vi "ER2007 Test Panel.vi"() -> ()   [LabVIEW 2013]
uses:
  Controls/Global ER2007.vi
panel:
  in  "Defeated":bool
  in  "Sim":bool
  in  "Radio Cell Selects":T1(ring)
  out "Clock":string
  in  "Reset DAQ":bool
  out "VPA Err":bool
  out "Elap-T":string="Lapsed Hrs"
  out "Last-T":string="Time"
  out "ProdVol":string="Produced Vol (cc)"
  out "Dnstrm-P":string="Downstrm P (psi)"
  out "Delta-P":string="Delta-P (psi)"
  out "Pore-P":string="Pore P (psi)"
  out "Conf-P":string="Confining P (psi)"
  out "TB":string="T-B (°C)"
  out "TA":string="T-A (°C)"
  out "FF23":string="FF 2-3"
  out "ER23":string="E-R 2-3 (Ohm-m)"
  out "ER14":string="E-R 1-4 (Ohm-m)"
  out "ER13":string="E-R 1-3 (Ohm-m)"
  out "ER12":string="E-R 1-2 (Ohm-m)"
  out "SampID":string="Sample ID"
  out "Cell #":string="Cell #"
  out "Status":string="Status"
  out "Other PC Busy":bool
  out "GCD Reset":bool
  out "Delta P (psi)":dbl[](array[numeric]) format="%.2f"
  out "Pc-d(psig)":dbl[](array[numeric])
  in  "TakePt":bool
  out "System Error":bool
  out "Refresh":bool
  out "SetupCell":i32
  out "GCDCell":i32
  out "SelCell":i32
  out "C5-Status":bool caption="VPA"
  out "C4-Status":bool caption="Manual"
  out "C3-Status":bool caption="VPA"
  out "C2-Status":bool caption="Manual"
  out "C1-Status":bool caption="Manual"
  in  "GCD Progress Titles":string="Initialize  Main Eng  Determ-R  Final Vals Close HP Close NAII"
  out "GCD Prog":bool[](array[boolean])
  out "Selected Data Cell":i32
  out "Cell Data Idx":i32
  out "Cur Time":dbl
  out "Schd Times":dbl[](array[numeric])
  out "GCD Err":bool
  out "GCD Busy":bool
  out "A/D Err":bool
  out "DAQ Run":bool
  in  "Radio Cell Selects":T2(radio)
  in  "Utilities":bool
  out "F 2-3":dbl[](array[numeric])=[6.3872, 0.0, 5.0918, 5.4196, 0.0, 5.8365, 5.8365, 0.0] format="%.2f"
  out "Cell":string[](array[string])=["Cell 1", "Cell 2", "Cell 3", "Cell 4", "Cell 5", "Cell 6B", "6B", "6C"]
  out "Copyrightl":string="Program ER2005, Version 1.00, DCI Inc, Copyright 2005, All Rights Reserved"
  out "Disp Pv (ml)":dbl[](array[numeric])=[12.345, 0.0, 2.509, 2.736, 0.0, 1.983, 508.0, 0.0] format="%.2f"
  in  "CurVals":bool
  in  "History":bool
  in  "Setup":bool
  in  "Stop":bool
  out "Lapsed Hrs":dbl[](array[numeric])=[789.0, 0.0, 107.6, 105.8, 0.0, 51.2, 51.2, 0.0] format="%.1f"
  out "Time":timestamp[](array[timestamp])=[timestamp(3199615260.25 s since 1904-01-01), timestamp(3199586400.25 s since 1904-01-01), timestamp(3199635000.25 s since 1904-01-01), timestamp(3199623780.25 s since 1904-01-01), timestamp(3199586400.25 s since 1904-01-01), timestamp(3199669020.25 s since 1904-01-01), timestamp(3199669020.25 s since 1904-01-01), timestamp(3199586400.25 s since 1904-01-01)] format="%<%H:%M>T"
  out "Pc (psig)":dbl[](array[numeric])=[7492.0, 0.0, 3520.0, 3488.0, 0.0, 508.0, 508.0, 0.0]
  out "NOP (psig)":dbl[](array[numeric])=[10058.0, 0.0, 5018.0, 4993.0, 0.0, 904.0, 904.0, 0.0]
  out "T-B (°C)":dbl[](array[numeric])=[149.0, 23.0, 153.0, 149.0, 23.0, 150.0, 150.0, 22.0] format="%.1f"
  out "T-A (°C)":dbl[](array[numeric])=[152.0, 22.0, 150.0, 147.0, 23.0, 151.0, 151.0, 22.0] format="%.1f"
  out "ER 2-3":dbl[](array[numeric])=[6.3872, 0.0, 5.0918, 5.4196, 0.0, 5.8365, 5.8365, 0.0] format="%.3f"
  out "ER 1-4":dbl[](array[numeric])=[6.1683, 0.0, 5.0447, 5.2485, 0.0, 5.6703, 5.6703, 0.0] format="%.3f"
  out "ER 1-3":dbl[](array[numeric])=[6.0887, 0.0, 4.9169, 5.2753, 0.0, 5.5338, 5.5338, 0.0] format="%.3f"
  out "ER 1-2":dbl[](array[numeric])=[6.7304, 0.0, 5.356, 5.9831, 0.0, 6.0646, 6.0646, 0.0] format="%.3f"
  out "Sample ID":string[](array[string])=["Sample #1", "", "Sample #3", "Sample #4", "", "Sample #6", "Sample #6", "  "]
  out "Status":bool[](array[boolean])=[FALSE, FALSE, FALSE, FALSE, FALSE, FALSE, TRUE, FALSE]
  # "Test Data"
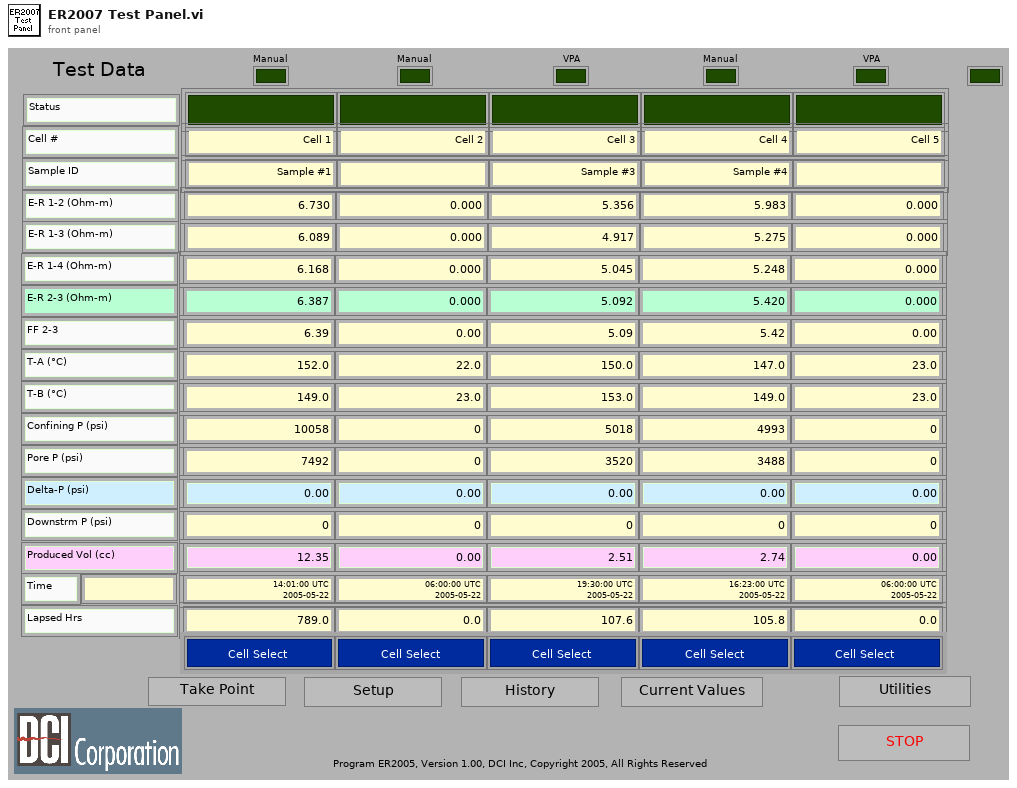
[diagram p1: front panel]
types:
  T1 = enum32{"No Selection", "CS 1", "CS 2", "CS 3", "CS 4", "CS 5", "CS 6"}
  T2 = enum32{"No Selection", "CS 1", "CS 2", "CS 3", "CS 4", "CS 5"}
  T3 = cluster{"PageTitle":string, "NumLines":i32, "ChlNum":string[], "ChlDesc":string[], "ChlUnits":string[], "ChlZero":sgl[], "ChlFactor":sgl[], "ChlConfig":u16[]}[]
  T4 = enum16{"Cell 1", "Cell 2", "Cell 3", "Cell 4", "Cell 5", "Cell 6A", "Cell 6B", "Cell 6C"}[]
  T5 = cluster{"CurCell":i32, "Cell Data":cluster{"Cell ID":i32, "Cell Status":enum16{"Inactive", "Setup", "Active", "Done"}, "Project":string, "Sample #":string, "Rock Type":string, "Fluid Pair":string, "Rw":dbl, "Rw Temp":dbl, "Length":dbl, "Diameter":dbl, "Porosity":dbl, "Permeability":dbl, "4P":bool, "ElectSpace":dbl, "Frequency":dbl, "Amplitude":dbl, "DAQ Period":u32, "DAQ Units":u16, "Start Time":dbl, "Next Time":dbl, "Datafile":path, "Last Pore Vol":dbl, "Last Pore Xdcr":enum16{"<none>", "Lo Range", "Hi Range"}, "Last Resistor":enum16{"<none>", "Resistor 1", "Resistor 2", "Resistor 3", "Resistor 4", "Resistor 5", "Resistor 6"}, "CurData":dbl[][], "Comment":string}[]}
  T6 = cluster{"Cell ID":i32, "Cell Status":enum16{"Inactive", "Setup", "Active", "Done"}, "Project":string, "Sample #":string, "Rock Type":string, "Fluid Pair":string, "Rw":dbl, "Rw Temp":dbl, "Length":dbl, "Diameter":dbl, "Porosity":dbl, "Permeability":dbl, "4P":bool, "ElectSpace":dbl, "Frequency":dbl, "Amplitude":dbl, "DAQ Period":u32, "DAQ Units":u16, "Start Time":dbl, "Next Time":dbl, "Datafile":path, "Last Pore Vol":dbl, "Last Pore Xdcr":enum16{"<none>", "Lo Range", "Hi Range"}, "Last Resistor":enum16{"<none>", "Resistor 1", "Resistor 2", "Resistor 3", "Resistor 4", "Resistor 5", "Resistor 6"}, "CurData":dbl[][], "Comment":string}[]
  T7 = cluster{"Cell ID":i32, "Cell Status":enum16{"Inactive", "Setup", "Active", "Done"}, "Project":string, "Sample #":string, "Rock Type":string, "Fluid Pair":string, "Rw":dbl, "Rw Temp":dbl, "Length":dbl, "Diameter":dbl, "Porosity":dbl, "Permeability":dbl, "4P":bool, "ElectSpace":dbl, "Frequency":dbl, "Amplitude":dbl, "DAQ Period":u32, "DAQ Units":u16, "Start Time":dbl, "Next Time":dbl, "Datafile":path, "Last Pore Vol":dbl, "Last Pore Xdcr":enum16{"<none>", "Lo Range", "Hi Range"}, "Last Resistor":enum16{"<none>", "Resistor 1", "Resistor 2", "Resistor 3", "Resistor 4", "Resistor 5", "Resistor 6"}, "CurData":dbl[][], "Comment":string}
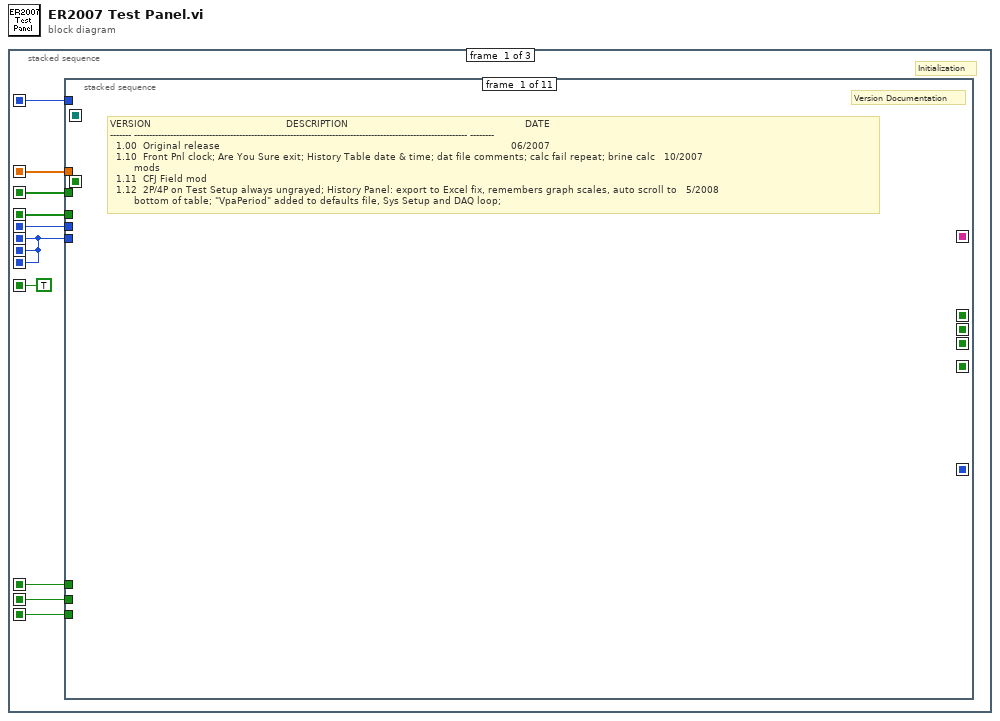
[diagram p0: block diagram]
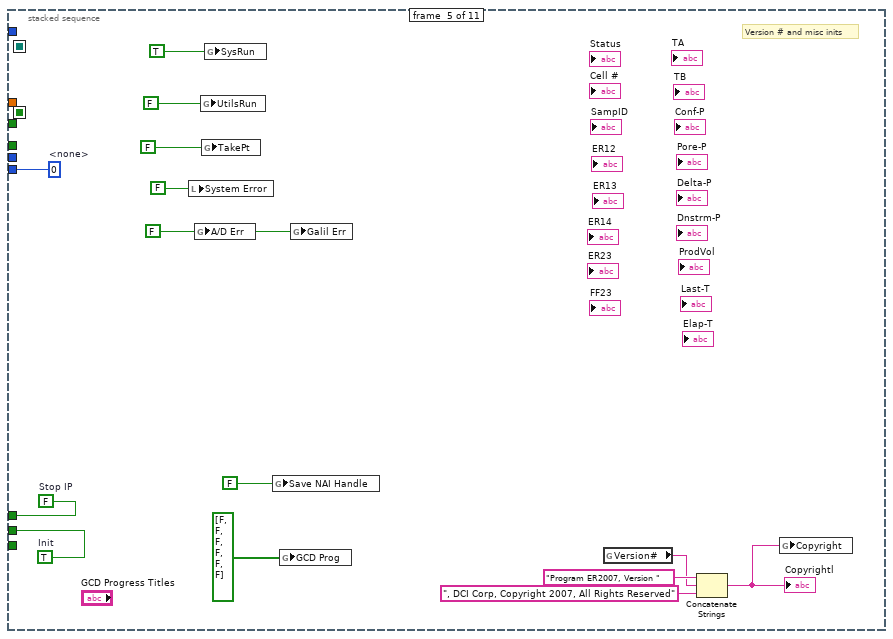
[diagram p5: hidden frame]
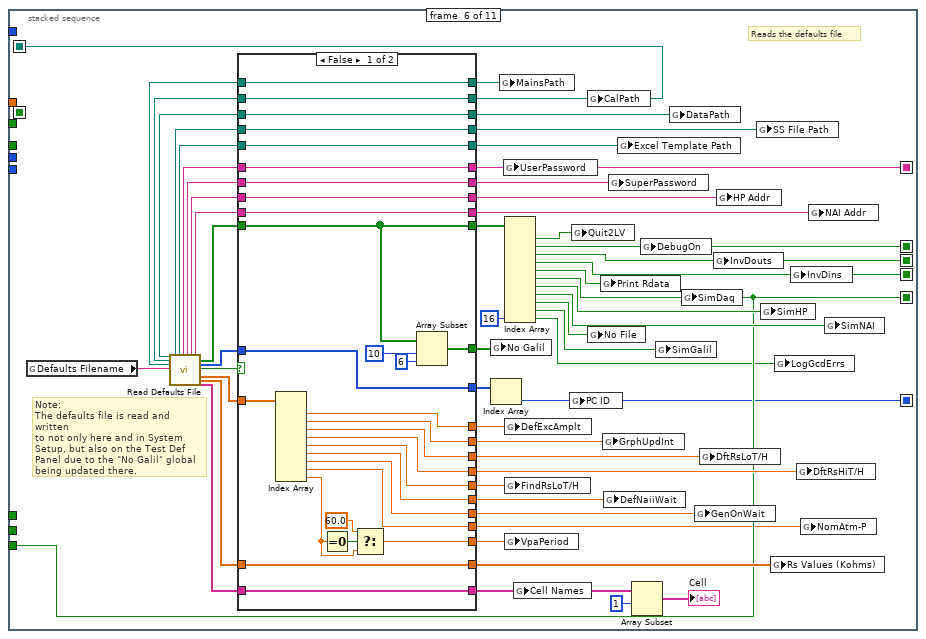
[diagram p6: hidden frame]
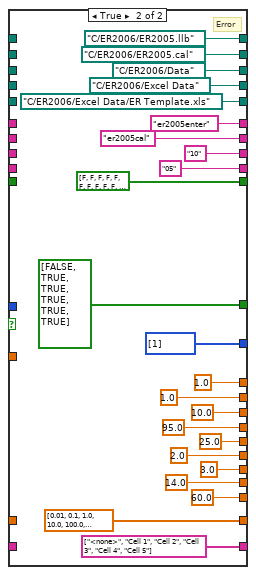
[diagram p7: hidden frame]
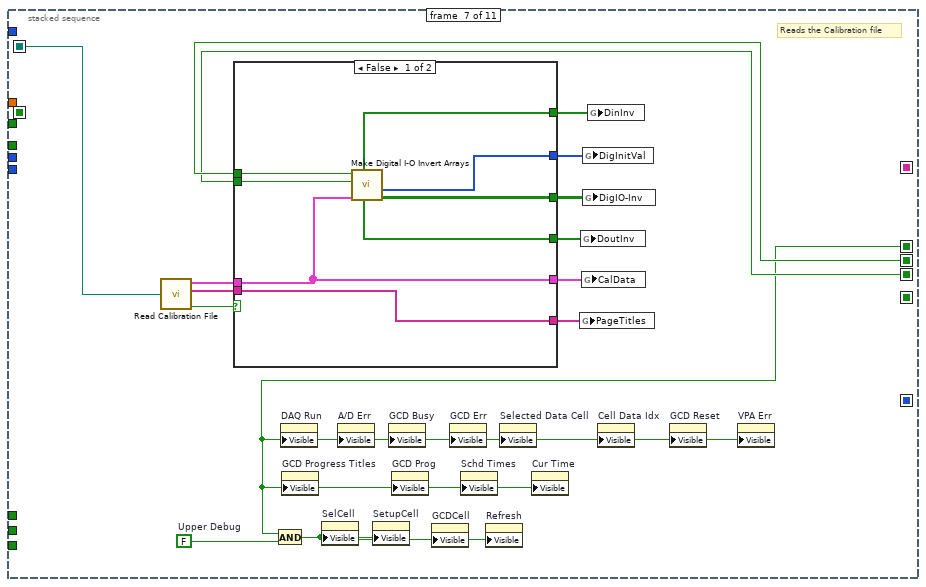
[diagram p8: hidden frame]
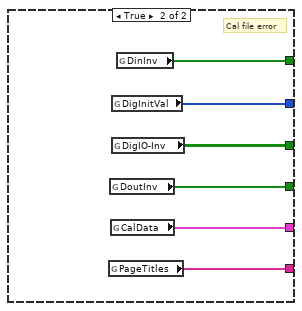
[diagram p9: hidden frame]
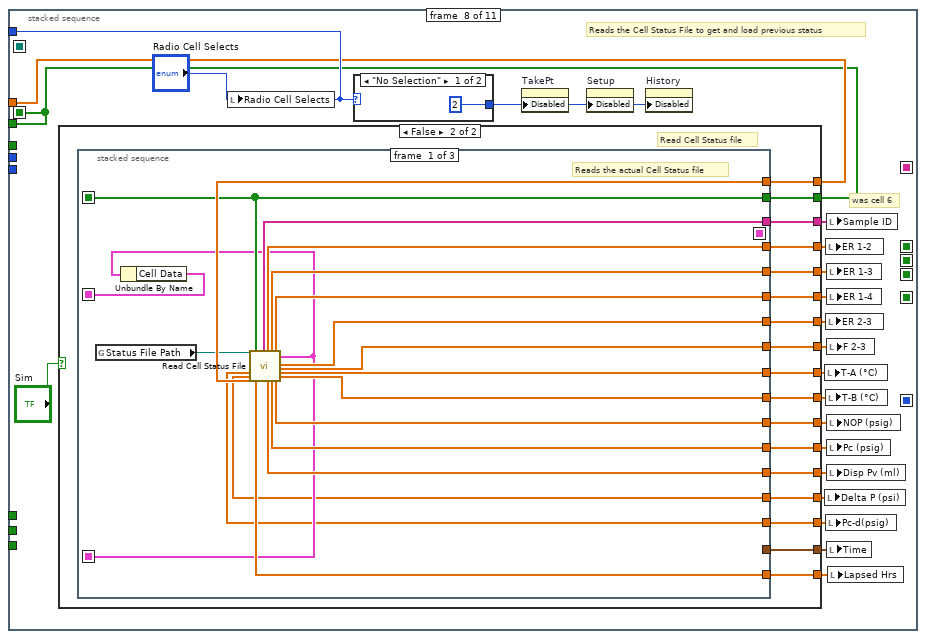
[diagram p10: hidden frame]
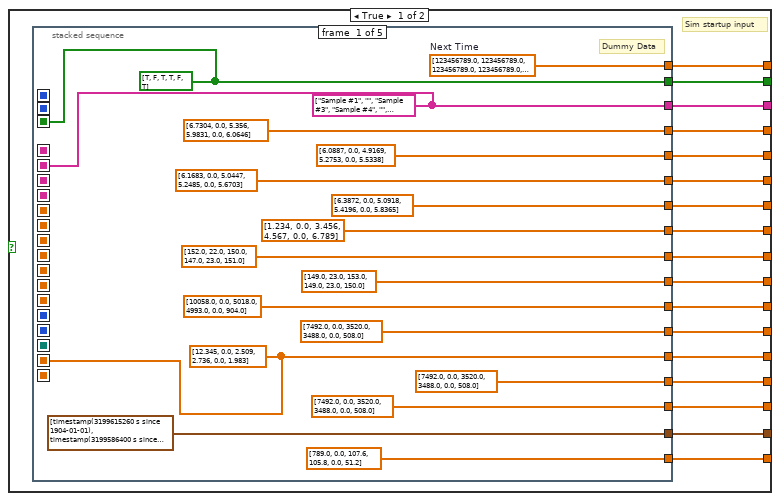
[diagram p11: hidden frame]
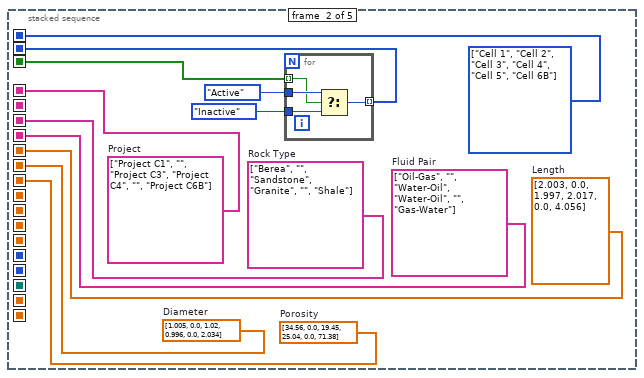
[diagram p12: hidden frame]
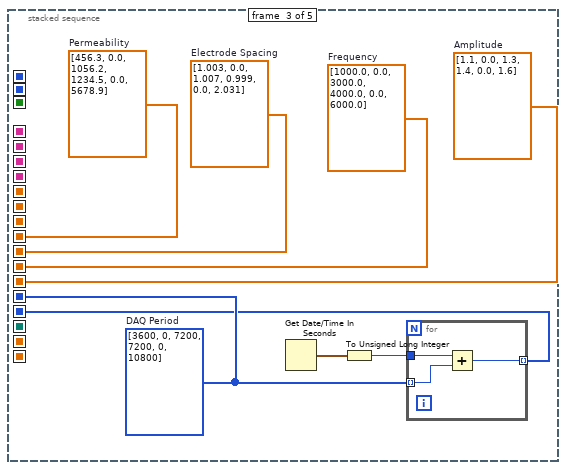
[diagram p13: hidden frame]
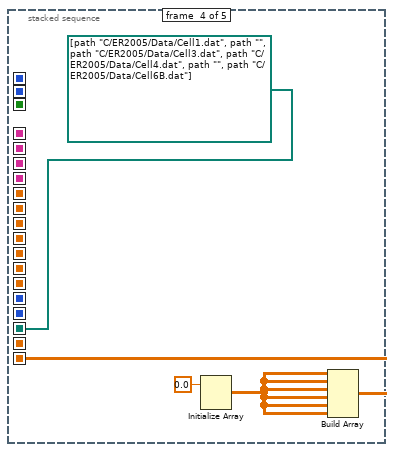
[diagram p14: hidden frame]
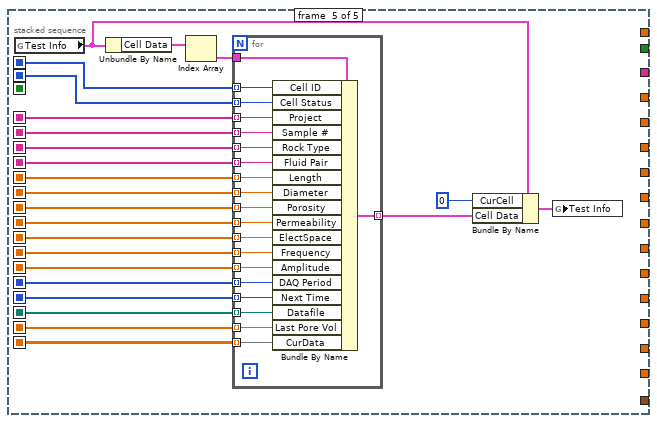
[diagram p15: hidden frame]
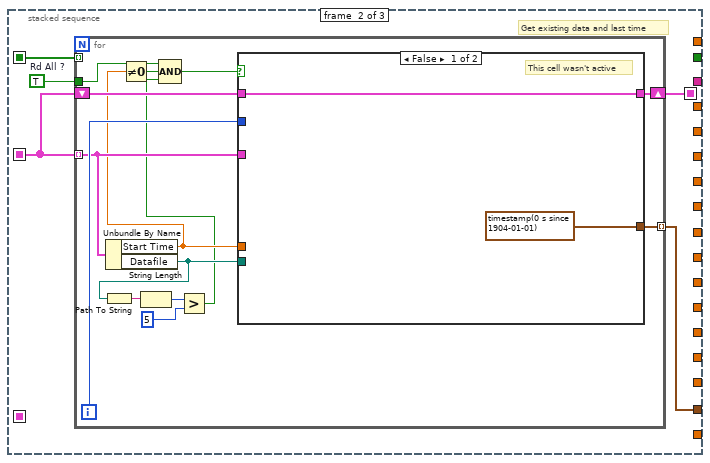
[diagram p16: hidden frame]
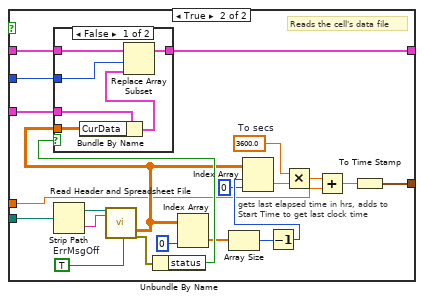
[diagram p17: hidden frame]
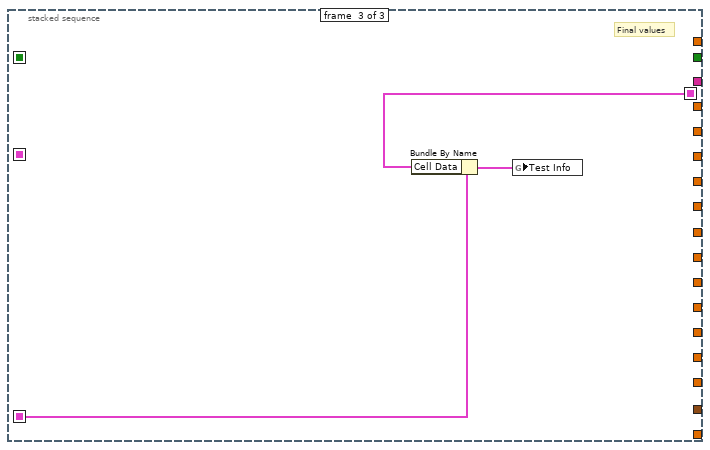
[diagram p19: hidden frame]
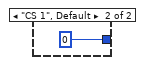
[diagram p20: hidden frame]
diagram:
  n1 = stacked-sequence {
    seq-local: [w10 _ _] -> [_ w451 _]
    seq-local: [w9 _ _] -> [_ w450 _]
    seq-local: [w8 _ _] -> [_ w449 _]
    seq-local: [w7 _ _] -> [_ w448 _]
    seq-local: [w6 _ _] -> [_ w447 _]
    seq-local: [w5 _ _] -> [_ w445 _]
    seq-local: [w5 _ _] -> [_ w446 _]
    seq-local: [w5 _ _] -> [_ w444 _]
    seq-local: [TRUE _ _] -> [_ w443 _]
    seq-local: [w3 _ _] -> [_ w442 w1331]
    seq-local: [w2 _ _] -> [_ w441 _]
    seq-local: [w1 _ _] -> [_ w440 _]
    frame #0 {
      # "Initialization"
      n2 = stacked-sequence {
        seq-local: [_ _ _ _ _ w58 _ _ _ _ _] -> [_ _ _ _ _ _ w140 _ _ _ _]
        seq-local: [_ _ _ _ _ w57 _ _ _ _ _] -> [_ _ _ _ _ _ _ _ _ _ _]
        seq-local: [_ _ _ _ _ w52 _ _ _ _ _] -> [_ _ _ _ _ _ w142 _ _ _ _]
        seq-local: [_ _ _ _ _ w53 _ _ _ _ _] -> [_ _ _ _ _ _ w141 _ _ _ _]
        seq-local: [_ _ _ _ _ _ _ w162 _ _ _] -> [_ _ _ _ _ _ _ _ _ w391 _]
        seq-local: [_ _ _ _ _ w50 _ _ _ _ _] -> [_ _ _ _ _ _ w131 _ _ _ _]
        seq-local: [_ _ _ _ _ w35 _ _ _ _ _] -> [_ _ _ _ _ _ _ _ w383 _ _]
        seq-local: [_ _ _ _ _ w34 _ _ _ _ _] -> [_ _ _ _ _ _ _ _ w380 _ _]
        tunnel: [_ _ _ _ _ _ _ w164 _ _ _] -> w10
        tunnel: [_ _ _ _ _ _ _ "Radio Cell Selects" _ _ _] -> w9
        tunnel: [_ _ _ _ w22 _ _ _ _ _ _] -> w8
        tunnel: [_ _ _ _ _ _ _ w162 _ _ _] -> w7
        tunnel: [_ _ _ _ _ _ _ _ _ w388 _] -> w6
        tunnel: [_ _ _ _ w13 _ _ _ _ _ _] -> w5
        tunnel: [_ _ _ _ _ w35 _ _ _ _ _] -> w3
        tunnel: [_ _ _ _ _ _ _ _ w379 _ _] -> w2
        tunnel: [_ _ _ _ w11 _ _ _ _ _ _] -> w1
        frame #0 {
          # "VERSION                                             DESCRIPTION                                                           DATE \n------- --------------------------------------------------------------------------------------------------------------- --------\n  1.00  Original release                                                                                                 06/2007\n  1.10  Front Pnl clock; Are You Sure exit; History Table date & time; dat file comments; calc fail repeat; brine calc   10/2007\n        mods\n  1.11  CFJ Field mod\n  1.12  2P/4P on Test Setup always ungrayed; History Panel: export to Excel fix, remembers graph scales, auto scroll to   5/2008\n        bottom of table; \"VpaPeriod\" added to defaults file, Sys Setup and DAQ loop;"
          # "Version Documentation"
        }
        frame #1 {
          # "New Cell Status Format\n\n[GenInfo]\nTitle=\"Cell Status Data File\"\nVersion=1.00\nLast Write=8/7/2005\nCurCell=\"2\"\n*NumCells=\"5\"\n[Cell 1 Status]\nCell ID=\"Cell 1\"\nStatus=Inactive\nProject=\"Project Cell 1\"\nSample ID=\"Sample #1\"\nRock Type=Granite\nFluid Pair=\"Brine & Air\"\nRw=11.000000\nRw Temp=22.000000\nLength=5.080000\nDiameter=2.540000\nPorosity=33.000000\nPermeability=8.000000\n2P/4P=4P\nElect Spacing=2.540000\nFrequency=1000.000000\nAmplitude=1.000000\nDAQ Period=1\nDAQ Units=Hrs\nStart Time=3205931570.670000\nNext Time=3205935200.670000\nFilename=\"C:\\\\ER2005\\\\Data\\\\Cell 1 Data.dat\"\nPore Volume=1.000000\n*Pore Transducer=\"Lo Range\"\nLast Resistor=\"Resistor 5\"\nER 1-2=4023.631104\nER 1-3=2923.760010\nER 1-4=3594.040039\nER 2-3=2434.518066\nFF 2-3=235.399994\nTemp A=24.799999\nTemp B=24.799999\nConf Press=5.000000\nPore Press=2.330000\nDelta-Press=\nPore-Down=\n[Cell 2 Status]"
          # "New Data File Format-Data Line\n\n                        Reals\nCol #  Process Variable Col #\n----- ----------------- -----\n  1   Point Flag\n  2   Point Date\n  3   Point Time\n  4   Elapsed Time (hrs)   1\n  5   ER 1-2               2\n  6   ER 1-3               3\n  7   ER 1-4               4\n  8   ER 2-3               5\n  9   F 2-3                6\n 10   T-A                  7\n 11   T-B                  8\n 12   Conf P (ER2005 NOP)  9\n 13   Pore P (ER2005 Pc)  10\n 14   Delta-P             11\n 15   Downstrm P (Pc-d)   12\n 16   Produced Vol        13\n 17   C14                 14\n 18   C23                 15\n 19   Comment"
          # "Dynamically Launched vi's:                     Other Required Files: simply copy them to System32\n-----------------------------------------      --------------------------------------------------------\nER2007 Are You Sure Popup Panel.vi             C:\\Windows\\System32\\instrsup.dll - used by NAII vi's\nER2007 Background DAQ Loop.vi                  C:\\Windows\\System32\\NAI2250.dll - used by NAII vi's\nER2007 Calibration Panel.vi                    C:\\Windows\\System32\\DMC32.dll - used by Galil vi's\nER2007 Current Values Panel.vi                 \nER2007 Data History Panel.vi\nER2007 Get Cell Data.vi\nER2007 Maintenance Panel.vi\nER2007 Password Popup Panel.vi\nER2007 System Setup Panel.vi\nER2007 Take Data Popup Panel.vi\nER2007 Test Definition Panel.vi\nER2007 Utilities Menu Panel.vi\nC:\\Program Files\\National Instruments\\LabVIEW 7.1\\vi.lib\\\n (cont)  addons\\_office\\_exclsub.llb\\_Excel Dynamic VIs.vi"
          # "Data File Format-Header\n\nStart Date\nStart Time\nFilename\nProject\nSample ID\nRock Type\nFluid Pair\nRw\nRt\nFrequency\nAmplitude\nDAQ Period (mins)\nLength\nDiameter\nPorosity\nPermeability\nElectrode Spacing"
          # "The arrays and controls on the front panel are a Arial Bold at 20 pt (18 pt plus two cntrl+)\nThe front panel color (matches Logo): Hue-135; Sat-43; Lum-109; Red-95; Grn-121; Blue-137"
          # "Notes and misc initilization"
        }
        frame #2 {
          # "More notes: Device 1 hardware assignments"
          # "PCI-6220 PV Assignments\n\n                      Connector 0\n        DIGITAL OUTS                ANALOG INS\n----------------------------  ------------------------\nP0.0    Shunt NOP1/Pc1A       AI 0    NOP1\nP0.1    SCL1                  AI 1    TC1A\nP0.2    SCL2                  AI 2    TC1B\nP0.3    Shunt Pc1B            AI 3    Pc1B\nP0.4    Auto Enable           AI 4    <spare>\nP0.5    RSCL1                 AI 5    <spare>\nP0.6    <spare>               AI 6    <spare>\nP0.7    RSCL2                 AI 7    <spare>\n\nP1.0    RSCL3                 AI 8    Pc1A\nP1.1    YCL1                  AI 9    CJ1A\nP1.2    YCL2                  AI 10   CJ1B\nP1.3    YCL3                  AI 11   <spare>\nP1.4    YCL4                  AI 12   <spare>\nP1.5    <spare>               AI 13   <spare>\nP1.6    Lockout               AI 14   <spare>\nP1.7    <spare>               AI 15   <spare>\n\n        DIGITAL INS\n----------------------------\nP2.0    <spare>\nP2.1    <spare>\nP2.2    <spare>\nP2.3    <spare>\nP2.4    <spare>\nP2.5    <spare>\nP2.6    <spare>\nP2.7    <spare>"
        }
        frame #3 {
          # "GPIB Setup and Operational Notes\n\n1) Using MAX, setup the PC #1 GPIB board as System\n   Controller with a primary address of 1.  Setup the\n   PC #2 GBIP board as a Non-System Controller with a\n   primary address of 2.\n2) Initialization is still a problem\n3) When PC #1 is active (taking a point), it asserts\n   Send IFC to clear the bus and take charge.  After\n   it has completed, it returns CIC control to PC #2\n   using PassControl."
          # "PCI-6224 PV Assignments By Connector Number\n\n                      Connector 1\n        DIGITAL OUTS                ANALOG INS\n----------------------------  ------------------------\nP0.8    Shunt NOP4/Pc4A       AI 16   NOP4\nP0.9    <spare>               AI 17   TC4A\nP0.10   <spare>               AI 18   TC4B\nP0.11   Shunt NOP5/Pc4B       AI 19   Pc4B\nP0.12   <spare>               AI 20   <spare>\nP0.13   Shunt Pc5A/Pc5B       AI 21   Pc5A\nP0.14   <spare>               AI 22   TC5A\nP0.15   <spare>               AI 23   TC5B\n\n                              AI 24   Pc4A\n                              AI 25   CJ4A\n                              AI 26   CJ4B\n                              AI 27   NOP5\n                              AI 28   <spare>\n                              AI 29   Pc5B\n                              AI 30   CJ5A\n                              AI 31   CJ5B"
          # "PCI-6224 PV Assignments By Connector Number\n\n                      Connector 0\n        DIGITAL OUTS                ANALOG INS\n----------------------------  ------------------------\nP0.0    Shunt NOP2/Pc2A       AI 0    NOP2\nP0.1    <spare>               AI 1    TC2A\nP0.2    <spare>               AI 2    TC2B\nP0.3    Shunt NOP3/Pc2B       AI 3    Pc2B\nP0.4    <spare>               AI 4    <spare>\nP0.5    Shunt Pc3A/Pc3B       AI 5    Pc3A\nP0.6    <spare>               AI 6    TC3A\nP0.7    <spare>               AI 7    TC3B\n\nP1.0    <spare>               AI 8    Pc2A\nP1.1    <spare>               AI 9    CJ2A\nP1.2    <spare>               AI 10   CJ2B\nP1.3    <spare>               AI 11   NOP3\nP1.4    <spare>               AI 12   <spare>\nP1.5    <spare>               AI 13   Pc3A\nP1.6    <spare>               AI 14   CJ3A\nP1.7    <spare>               AI 15   CJ3B\n\n        DIGITAL INS\n----------------------------\nP2.0    Busy 1\nP2.1    Busy 2\nP2.2    <spare>\nP2.3    <spare>\nP2.4    <spare>\nP2.5    <spare>\nP2.6    <spare>\nP2.7    <spare>"
          # "More notes: Device 2 hardware assignments"
        }
        frame #4 {
          w11 = FALSE  # Stop IP
          w12 = FALSE ("A/D Err")
          w13 = 0  # <none>
          w22 = TRUE  # Init
          # "Version # and misc inits"
          n3 = local write "System Error"(FALSE ("System Error")) -> ()
          n4 = global write "Global ER2007.vi" "A/D Err"(w12) -> ()
          n5 = global write "Global ER2007.vi" "UtilsRun"(FALSE ("UtilsRun")) -> ()
          n6 = global write "Global ER2007.vi" "TakePt"(FALSE ("New Setup")) -> ()
          n7 = global write "Global ER2007.vi" "SysRun"(TRUE ("SysRun")) -> ()
          n8 = global write "Global ER2007.vi" "Save NAI Handle"(FALSE ("Save NAI Handle")) -> ()
          n9 = global write "Global ER2007.vi" "GCD Prog"(bool[] [FALSE, FALSE, FALSE, FALSE, FALSE, FALSE] ("GCD Prog")) -> ()
          n10 = global write "Global ER2007.vi" "Galil Err"(w12) -> ()
          n11 = global read "Global ER2007.vi" "Version#"() -> (w20:string)
          n12 = Concatenate Strings("Program ER2007, Version " ("Substring"), w20, ", DCI Corp, Copyright 2007, All Rights Reserved" ("Substring")) -> (w19:string)
          "Copyrightl" <- w19
          n13 = global write "Global ER2007.vi" "Copyright"(w19) -> ()
        }
        frame #5 {
          # "Note:\nThe defaults file is read and written\nto not only here and in System\nSetup, but also on the Test Def\nPanel due to the \"No Galil\" global\nbeing updated there."
          # "Reads the defaults file"
          n14 = global read "Global ER2007.vi" "Defaults Filename"() -> (w37:string)
          n15 = call "Read Defaults File.vi"("Filename"=w37) -> ("DirPath3"=w73:path, "DirPath2"=w74:path, "DirPath1"=w75:path, "DirPath4"=w66:path, "DirPath5"=w65:path, "String1"=w72:string, "String2"=w71:string, "String3"=w69:string, "String4"=w68:string, "BooleanArray"=w77:bool[], "IntegerArray1"=w64:i32[], "ErrOut"=w78:bool, "RealArray1"=w70:dbl[], "RealArray2"=w67:dbl[], "StringArray"=w36:string[])  [unwired: 12 out]
          n16 = case shown="False" w78 {
            tunnel: w77 -> [w86 _]
            tunnel: [w86 bool[] [FALSE, FALSE, FALSE, FALSE, FALSE, FALSE, FALSE, FALSE, FALSE, FALSE, FALSE, FALSE] ("BooleanArray")] -> w76
            tunnel: [w107 path "C:/ER2006/ER2005.llb" ("DirPath1")] -> w59
            tunnel: w75 -> [w107 _]
            tunnel: [w106 path "C:/ER2006/ER2005.cal" ("DirPath2")] -> w58
            tunnel: w74 -> [w106 _]
            tunnel: [w105 path "C:/ER2006/Data" ("DirPath3")] -> w62
            tunnel: w73 -> [w105 _]
            tunnel: [w104 "er2005enter" ("String1")] -> w57
            tunnel: w72 -> [w104 _]
            tunnel: [w103 "er2005cal" ("String2")] -> w56
            tunnel: w71 -> [w103 _]
            tunnel: w70 -> [w100 _]
            tunnel: [w102 "10" ("String3")] -> w55
            tunnel: w69 -> [w102 _]
            tunnel: [w101 "05" ("String4")] -> w54
            tunnel: w68 -> [w101 _]
            tunnel: [w99 1.0] -> w45
            tunnel: [w98 1.0] -> w44
            tunnel: [w97 10.0] -> w43
            tunnel: [w96 95.0] -> w42
            tunnel: w67 -> [w95 _]
            tunnel: [w95 dbl[] [0.01, 0.1, 1.0, 10.0, 100.0, 1000.0] ("RealArray2")] -> w38
            tunnel: [w94 25.0] -> w41
            tunnel: [w93 path "C:/ER2006/Excel Data" ("SS File Path")] -> w61
            tunnel: w66 -> [w93 _]
            tunnel: [w92 2.0] -> w40
            tunnel: [w91 3.0] -> w39
            tunnel: [w90 path "C:/ER2006/Excel Data/ER Template.xls" ("Excel Template Path")] -> w60
            tunnel: w65 -> [w90 _]
            tunnel: w64 -> [w89 _]
            tunnel: [w89 i32[] [1] ("IntegerArray1")] -> w63
            tunnel: w36 -> [w88 _]
            tunnel: [w88 string[] ["<none>", "Cell 1", "Cell 2", "Cell 3", "Cell 4", "Cell 5"] ("StringArray")] -> w31
            tunnel: [w87 14.0 ("NomAtm-P")] -> w32
            tunnel: [w83 bool[] [FALSE, TRUE, TRUE, TRUE, TRUE, TRUE]] -> w28
            tunnel: [w79 60.0 ("VpaPeriod")] -> w25
            frame False {
              n17 = Index Array(array=w100) -> (element #1=w99:dbl, element #2=w98:dbl, element #3=w97:dbl, element #4=w96:dbl, element #5=w94:dbl, element #6=w92:dbl, element #7=w91:dbl, element #8=w87:dbl, element #9=w80:dbl)  [unwired: 9 in]
              n18 = Equal To 0?(x=w80) -> (x = 0?=w82:bool)
              n19 = Select(t=60.0, s=w82, f=w80) -> (s? t:f=w79:dbl)
              n20 = Array Subset(array=w86, index=10, length=6) -> (w83:bool[])
            }
            frame True {
              # "Error"
            }
          }
          n21 = global write "Global ER2007.vi" "No Galil"(w28) -> ()
          n22 = Index Array(array=w63) -> (element=w34:i32)  [unwired: 1 in]
          n23 = global write "Global ER2007.vi" "MainsPath"(w59) -> ()
          n24 = global write "Global ER2007.vi" "UserPassword"(w57) -> ()
          n25 = Index Array(array=w76, index #11=16 ("index")) -> (element #1=w51:bool, element #2=w50:bool, element #3=w52:bool, element #4=w53:bool, element #5=w49:bool, element #6=w35:bool, element #7=w48:bool, element #8=w47:bool, element #9=w46:bool, element #10=w33:bool, element #11=w26:bool)  [unwired: 10 in]
          n26 = global write "Global ER2007.vi" "DefExcAmplt"(w45) -> ()
          n27 = global write "Global ER2007.vi" "FindRsLoT/H"(w41) -> ()
          n28 = global write "Global ER2007.vi" "VpaPeriod"(w25) -> ()
          n29 = global write "Global ER2007.vi" "Cell Names"(w31) -> ()
          n30 = global write "Global ER2007.vi" "PC ID"(w34) -> ()
          n31 = global write "Global ER2007.vi" "Quit2LV"(w51) -> ()
          n32 = global write "Global ER2007.vi" "CalPath"(w58) -> ()
          n33 = global write "Global ER2007.vi" "No File"(w46) -> ()
          n34 = global write "Global ER2007.vi" "Print Rdata"(w49) -> ()
          n35 = global write "Global ER2007.vi" "GrphUpdInt"(w44) -> ()
          n36 = global write "Global ER2007.vi" "DefNaiiWait"(w40) -> ()
          n37 = global write "Global ER2007.vi" "SuperPassword"(w56) -> ()
          n38 = global write "Global ER2007.vi" "Excel Template Path"(w60) -> ()
          n39 = Array Subset(array=w31, index=1) -> (→"Cell":string[])  [unwired: 1 in]
          n40 = global write "Global ER2007.vi" "DebugOn"(w50) -> ()
          n41 = global write "Global ER2007.vi" "SimGalil"(w33) -> ()
          n42 = global write "Global ER2007.vi" "DataPath"(w62) -> ()
          n43 = global write "Global ER2007.vi" "SimDaq"(w35) -> ()
          n44 = global write "Global ER2007.vi" "GenOnWait"(w39) -> ()
          n45 = global write "Global ER2007.vi" "DftRsLoT/H"(w43) -> ()
          n46 = global write "Global ER2007.vi" "InvDouts"(w52) -> ()
          n47 = global write "Global ER2007.vi" "HP Addr"(w55) -> ()
          n48 = global write "Global ER2007.vi" "SS File Path"(w61) -> ()
          n49 = global write "Global ER2007.vi" "SimHP"(w48) -> ()
          n50 = global write "Global ER2007.vi" "Rs Values (Kohms)"(w38) -> ()
          n51 = global write "Global ER2007.vi" "LogGcdErrs"(w26) -> ()
          n52 = global write "Global ER2007.vi" "InvDins"(w53) -> ()
          n53 = global write "Global ER2007.vi" "DftRsHiT/H"(w42) -> ()
          n54 = global write "Global ER2007.vi" "NomAtm-P"(w32) -> ()
          n55 = global write "Global ER2007.vi" "NAI Addr"(w54) -> ()
          n56 = global write "Global ER2007.vi" "SimNAI"(w47) -> ()
        }
        frame #6 {
          w138 = FALSE  # Upper Debug
          # "Reads the Calibration file"
          n57 = call "Read Calibration File.vi"("Filepath"=w140) -> ("CalData"=w144:T3, "PageTitles"=w143:string[], "ErrOut"=w145:bool)  [unwired: 1 in, 2 out]
          n58 = case shown="False" w145 {
            tunnel: w144 -> [w152 _]
            tunnel: w143 -> [w153 _]
            tunnel: [w152 w154] -> w133
            tunnel: [w153 w155] -> w132
            tunnel: w142 -> [w151 _]
            tunnel: w141 -> [w150 _]
            tunnel: [w149 w156] -> w134
            tunnel: [w148 w157] -> w135
            tunnel: [w147 w158] -> w136
            tunnel: [w146 w159] -> w137
            frame False {
              n59 = call "Make Digital I-O Invert Arrays.vi"("CalDataIn"=w152, "InvDins"=w150, "InvDouts"=w151) -> ("DIO-Inv"=w148:bool[][], "DoutInit"=w147:i32[], "DoutInv (1D)"=w149:bool[], "DinInv (1D)"=w146:bool[])  [unwired: 1 in, 4 out]
            }
            frame True {
              # "Cal file error"
              n60 = global read "Global ER2007.vi" "PageTitles"() -> (w155:string[])
              n61 = global read "Global ER2007.vi" "DoutInv"() -> (w156:bool[])
              n62 = global read "Global ER2007.vi" "CalData"() -> (w154:T3)
              n63 = global read "Global ER2007.vi" "DigInitVal"() -> (w158:i32[])
              n64 = global read "Global ER2007.vi" "DigIO-Inv"() -> (w157:bool[][])
              n65 = global read "Global ER2007.vi" "DinInv"() -> (w159:bool[])
            }
          }
          n66 = And(x=w131, y=w138) -> (x .and. y?=w139:bool)
          n67 = property on="DAQ Run" class="Bool (strict)"("Visible"=w131) -> ()  [unwired: 2 in, 2 out]
          n68 = property on="GCD Progress Titles" class="Str"("Visible"=w131) -> ()  [unwired: 2 in, 2 out]
          n69 = property on="SelCell" class="DigNum (strict)"("Visible"=w139) -> ()  [unwired: 2 in, 2 out]
          n70 = property on="A/D Err" class="Bool (strict)"("Visible"=w131) -> ()  [unwired: 2 in, 2 out]
          n71 = property on="SetupCell" class="DigNum (strict)"("Visible"=w139) -> ()  [unwired: 2 in, 2 out]
          n72 = property on="GCD Busy" class="Bool (strict)"("Visible"=w131) -> ()  [unwired: 2 in, 2 out]
          n73 = property on="GCD Prog" class="Arr (strict)"("Visible"=w131) -> ()  [unwired: 2 in, 2 out]
          n74 = property on="GCDCell" class="DigNum (strict)"("Visible"=w139) -> ()  [unwired: 2 in, 2 out]
          n75 = property on="GCD Err" class="Bool (strict)"("Visible"=w131) -> ()  [unwired: 2 in, 2 out]
          n76 = property on="Schd Times" class="Arr (strict)"("Visible"=w131) -> ()  [unwired: 2 in, 2 out]
          n77 = property on="Refresh" class="Bool (strict)"("Visible"=w139) -> ()  [unwired: 2 in, 2 out]
          n78 = property on="Selected Data Cell" class="DigNum (strict)"("Visible"=w131) -> ()  [unwired: 2 in, 2 out]
          n79 = property on="Cur Time" class="DigNum (strict)"("Visible"=w131) -> ()  [unwired: 2 in, 2 out]
          n80 = global write "Global ER2007.vi" "PageTitles"(w132) -> ()
          n81 = global write "Global ER2007.vi" "DoutInv"(w134) -> ()
          n82 = global write "Global ER2007.vi" "CalData"(w133) -> ()
          n83 = global write "Global ER2007.vi" "DigInitVal"(w136) -> ()
          n84 = global write "Global ER2007.vi" "DigIO-Inv"(w135) -> ()
          n85 = global write "Global ER2007.vi" "DinInv"(w137) -> ()
          n86 = property on="Cell Data Idx" class="DigNum (strict)"("Visible"=w131) -> ()  [unwired: 2 in, 2 out]
          n87 = property on="GCD Reset" class="Bool (strict)"("Visible"=w131) -> ()  [unwired: 2 in, 2 out]
          n88 = property on="VPA Err" class="Bool (strict)"("Visible"=w131) -> ()  [unwired: 2 in, 2 out]
        }
        frame #7 {
          # "was cell 6"
          # "Reads the Cell Status File to get and load previous status"
          n89 = case shown="False" "Sim" {
            tunnel: [w196 w292] -> w162
            tunnel: [w195 w304] -> w176
            tunnel: [w194 w303] -> w175
            tunnel: [w193 w302] -> w174
            tunnel: [w192 w301] -> w173
            tunnel: [w191 w300] -> w172
            tunnel: [w190 w299] -> w171
            tunnel: [w189 w298] -> w170
            tunnel: [w188 w297] -> w169
            tunnel: [w187 w296] -> w168
            tunnel: [w186 w295] -> w167
            tunnel: [w185 w294] -> w166
            tunnel: [w184 w293] -> w165
            tunnel: [w183 w291] -> w164
            tunnel: [w182 w290] -> w163
            tunnel: [w181 w289] -> w161
            tunnel: [w180 w288] -> w160
            frame True {
              # "Sim startup input"
              n90 = stacked-sequence {
                seq-local: [_ _ w229 _ _] -> [_ _ _ _ w251]
                seq-local: [_ _ w230 _ _] -> [_ _ _ _ w252]
                seq-local: [w211 _ _ _ _] -> [_ _ _ _ w264]
                seq-local: [_ w217 _ _ _] -> [_ _ _ _ w261]
                seq-local: [_ w216 _ _ _] -> [_ _ _ _ w260]
                seq-local: [_ w215 _ _ _] -> [_ _ _ _ w259]
                seq-local: [_ w214 _ _ _] -> [_ _ _ _ w258]
                seq-local: [_ _ w236 _ _] -> [_ _ _ _ w257]
                seq-local: [_ _ w235 _ _] -> [_ _ _ _ w256]
                seq-local: [_ _ w234 _ _] -> [_ _ _ _ w255]
                seq-local: [_ _ w233 _ _] -> [_ _ _ _ w254]
                seq-local: [w213 _ _ _ _] -> [_ _ _ _ w253]
                seq-local: [w212 _ _ _ _] -> [_ w223 _ _ _]
                seq-local: [_ w224 _ _ _] -> [_ _ _ _ w267]
                seq-local: [_ w220 _ _ _] -> [_ _ _ _ w265]
                seq-local: [_ w219 _ _ _] -> [_ _ _ _ w263]
                seq-local: [_ w218 _ _ _] -> [_ _ _ _ w262]
                seq-local: [_ _ _ path[] [path "C:/ER2005/Data/Cell1.dat", path "", path "C:/ER2005/Data/Cell3.dat", path "C:/ER2005/Data/Cell4.dat", path "", path "C:/ER2005/Data/Cell6B.dat"] _] -> [_ _ _ _ w250]
                seq-local: [_ _ _ w240 _] -> [_ _ _ _ w249]
                tunnel: [w212 _ _ _ _] -> w196
                tunnel: [w211 _ _ _ _] -> w195
                tunnel: [dbl[] [6.7304, 0.0, 5.356, 5.9831, 0.0, 6.0646] ("ER 1-2") _ _ _ _] -> w194
                tunnel: [dbl[] [6.0887, 0.0, 4.9169, 5.2753, 0.0, 5.5338] ("ER 1-3") _ _ _ _] -> w193
                tunnel: [dbl[] [6.1683, 0.0, 5.0447, 5.2485, 0.0, 5.6703] ("ER 1-4") _ _ _ _] -> w192
                tunnel: [dbl[] [6.3872, 0.0, 5.0918, 5.4196, 0.0, 5.8365] ("ER 2-3") _ _ _ _] -> w191
                tunnel: [dbl[] [152.0, 22.0, 150.0, 147.0, 23.0, 151.0] ("T-A") _ _ _ _] -> w190
                tunnel: [dbl[] [149.0, 23.0, 153.0, 149.0, 23.0, 150.0] ("T-B") _ _ _ _] -> w189
                tunnel: [dbl[] [10058.0, 0.0, 5018.0, 4993.0, 0.0, 904.0] ("Pc") _ _ _ _] -> w188
                tunnel: [dbl[] [7492.0, 0.0, 3520.0, 3488.0, 0.0, 508.0] ("Pp") _ _ _ _] -> w187
                tunnel: [w213 _ _ _ _] -> w186
                tunnel: [timestamp[] [timestamp(3199615260.25 s since 1904-01-01), timestamp(3199586400.25 s since 1904-01-01), timestamp(3199635000.25 s since 1904-01-01), timestamp(3199623780.25 s since 1904-01-01), timestamp(3199586400.25 s since 1904-01-01), timestamp(3199669020.25 s since 1904-01-01)] ("Last Time") _ _ _ _] -> w185
                tunnel: [dbl[] [789.0, 0.0, 107.6, 105.8, 0.0, 51.2] ("Run Time") _ _ _ _] -> w184
                tunnel: [w200 _ _ _ _] -> w183
                tunnel: [dbl[] [1.234, 0.0, 3.456, 4.567, 0.0, 6.789] ("F 2-3") _ _ _ _] -> w182
                tunnel: [dbl[] [7492.0, 0.0, 3520.0, 3488.0, 0.0, 508.0] ("Pp") _ _ _ _] -> w181
                tunnel: [dbl[] [7492.0, 0.0, 3520.0, 3488.0, 0.0, 508.0] ("Pp") _ _ _ _] -> w180
                frame #0 {
                  w200 = dbl[] [123456789.0, 123456789.0, 123456789.0, 123456789.0, 123456789.0, 123456789.0]  # Next Time
                  w213 = dbl[] [12.345, 0.0, 2.509, 2.736, 0.0, 1.983] ("Pore Vol")
                  w211 = string[] ["Sample #1", "", "Sample #3", "Sample #4", "", "Sample #6"] ("Sample ID")
                  w212 = bool[] [TRUE, FALSE, TRUE, TRUE, FALSE, TRUE] ("Run")
                  # "Dummy Data"
                }
                frame #1 {
                  w214 = dbl[] [34.56, 0.0, 19.45, 25.04, 0.0, 71.38]  # Porosity
                  w215 = dbl[] [1.005, 0.0, 1.02, 0.996, 0.0, 2.034]  # Diameter
                  w217 = string[] ["Oil-Gas", "", "Water-Oil", "Water-Oil", "", "Gas-Water"]  # Fluid Pair
                  w216 = dbl[] [2.003, 0.0, 1.997, 2.017, 0.0, 4.056]  # Length
                  w218 = string[] ["Berea", "", "Sandstone", "Granite", "", "Shale"]  # Rock Type
                  w219 = string[] ["Project C1", "", "Project C3", "Project C4", "", "Project C6B"]  # Project
                  w224 = T4 [enum."Cell 1", enum."Cell 2", enum."Cell 3", enum."Cell 4", enum."Cell 5", enum."Cell 6B"] items=["Cell 1", "Cell 2", "Cell 3", "Cell 4", "Cell 5", "Cell 6A", "Cell 6B", "Cell 6C"]
                  n91 = for {
                    tunnel: w223 -> [w226] mode=indexing
                    tunnel: enum16{"Inactive", "Setup", "Active", "Done"}."Active" ("Cell Status") -> [w228]
                    tunnel: enum16{"Inactive", "Setup", "Active", "Done"}."Inactive" ("Cell Status") -> [w227]
                    tunnel: [w225] -> w220 mode=indexing
                    n92 = Select(t=w228, s=w226, f=w227) -> (s? t:f=w225:enum16{"Inactive", "Setup", "Active", "Done"})
                  }
                }
                frame #2 {
                  w230 = u32[] [3600, 0, 7200, 7200, 0, 10800]  # DAQ Period
                  w233 = dbl[] [1.1, 0.0, 1.3, 1.4, 0.0, 1.6]  # Amplitude
                  w234 = dbl[] [1000.0, 0.0, 3000.0, 4000.0, 0.0, 6000.0]  # Frequency
                  w235 = dbl[] [1.003, 0.0, 1.007, 0.999, 0.0, 2.031]  # Electrode Spacing
                  w236 = dbl[] [456.3, 0.0, 1056.2, 1234.5, 0.0, 5678.9]  # Permeability
                  n93 = Get Date/Time In Seconds() -> (seconds since 1Jan1904=w232:timestamp)
                  n94 = To Unsigned Long Integer(number=w232) -> (unsigned 32bit integer=w231:u32)
                  n95 = for {
                    tunnel: w231 -> [w239]
                    tunnel: w230 -> [w238] mode=indexing
                    tunnel: [w237] -> w229 mode=indexing
                    n96 = Add(x=w239, y=w238) -> (x+y=w237:u32)
                  }
                }
                frame #3 {
                  n97 = Initialize Array(0.0 ("element")) -> (w241:dbl[][])  [unwired: 2 in]
                  n98 = Build Array(w241, w241, w241, w241, w241, w241) -> (w240:dbl[][][])
                }
                frame #4 {
                  n99 = global read "Global ER2007.vi" "Test Info"() -> (w245:T5)
                  n100 = Unbundle By Name(w245) -> ("Cell Data"=w247:T6)
                  n101 = Index Array(array=w247) -> (element=w248:T7)  [unwired: 1 in]
                  n102 = for {
                    tunnel: w248 -> [w287]
                    tunnel: w267 -> [w286] mode=indexing
                    tunnel: [w285] -> w266 mode=indexing
                    tunnel: w265 -> [w284] mode=indexing
                    tunnel: w264 -> [w283] mode=indexing
                    tunnel: w263 -> [w282] mode=indexing
                    tunnel: w262 -> [w281] mode=indexing
                    tunnel: w261 -> [w280] mode=indexing
                    tunnel: w260 -> [w279] mode=indexing
                    tunnel: w259 -> [w278] mode=indexing
                    tunnel: w258 -> [w277] mode=indexing
                    tunnel: w257 -> [w276] mode=indexing
                    tunnel: w256 -> [w275] mode=indexing
                    tunnel: w255 -> [w274] mode=indexing
                    tunnel: w254 -> [w273] mode=indexing
                    tunnel: w253 -> [w272] mode=indexing
                    tunnel: w252 -> [w271] mode=indexing
                    tunnel: w251 -> [w270] mode=indexing
                    tunnel: w250 -> [w269] mode=indexing
                    tunnel: w249 -> [w268] mode=indexing
                    n103 = Bundle By Name(cluster=w287, "Cell ID"=w286, "Cell Status"=w284, "Project"=w282, "Sample #"=w283, "Rock Type"=w281, "Fluid Pair"=w280, "Length"=w279, "Diameter"=w278, "Porosity"=w277, "Permeability"=w276, "ElectSpace"=w275, "Frequency"=w274, "Amplitude"=w273, "DAQ Period"=w271, "Next Time"=w270, "Datafile"=w269, "Last Pore Vol"=w272, "CurData"=w268) -> (w285:T7)
                  }
                  n104 = Bundle By Name(cluster=w245, "CurCell"=0, "Cell Data"=w266) -> (w246:T5)
                  n105 = global write "Global ER2007.vi" "Test Info"(w246) -> ()
                }
              }
            }
            frame False {
              # "Read Cell Status file"
              n106 = stacked-sequence {
                seq-local: [w308 _ _] -> [_ w327 _]
                seq-local: [w310 _ _] -> [_ w328 _]
                seq-local: [w309 _ _] -> [_ _ w376]
                seq-local: [_ w326 _] -> [_ _ w375]
                tunnel: [w323 _ _] -> w304
                tunnel: [w322 _ _] -> w303
                tunnel: [w321 _ _] -> w302
                tunnel: [w320 _ _] -> w301
                tunnel: [w319 _ _] -> w300
                tunnel: [w317 _ _] -> w299
                tunnel: [w316 _ _] -> w298
                tunnel: [w315 _ _] -> w297
                tunnel: [w314 _ _] -> w296
                tunnel: [w313 _ _] -> w295
                tunnel: [_ w324 _] -> w294
                tunnel: [w311 _ _] -> w293
                tunnel: [w310 _ _] -> w292
                tunnel: [w312 _ _] -> w291
                tunnel: [w318 _ _] -> w290
                tunnel: [w306 _ _] -> w289
                tunnel: [w305 _ _] -> w288
                frame #0 {
                  # "Reads the actual Cell Status file"
                  n107 = global read "Global ER2007.vi" "Status File Path"() -> (w307:path)
                  n108 = call "Read Cell Status File.vi"("FilePathIn"=w307) -> ("Pdn"=w305:dbl[], "Pdp"=w306:dbl[], "Next Time"=w312:dbl[], "Run Status"=w310:bool[], "Elapsed-T"=w311:dbl[], "SampID"=w323:string[], "ER 1-2"=w322:dbl[], "Pv"=w313:dbl[], "ER 1-3"=w321:dbl[], "Pp"=w314:dbl[], "ER 1-4"=w320:dbl[], "Pc"=w315:dbl[], "Test Info"=w309:T5, "ER 2-3"=w319:dbl[], "F 2-3"=w318:dbl[], "TA"=w317:dbl[], "TB"=w316:dbl[])  [unwired: 4 in, 6 out]
                  n109 = Unbundle By Name(w309) -> ("Cell Data"=w308:T6)
                }
                frame #1 {
                  w325 = TRUE  # Rd All ?
                  # "Get existing data and last time"
                  n110 = for {
                    tunnel: w327 -> [w337] mode=indexing
                    tunnel: w328 -> [_] mode=indexing
                    shift-right: [w341] -> w326
                    shift-left: w327 -> [w342]
                    tunnel: [w339] -> w324 mode=indexing
                    tunnel: w325 -> [w331]
                    i -> [w340]
                    n111 = Unbundle By Name(w337) -> ("Start Time"=w330:dbl, "Datafile"=w335:path)
                    n112 = Path To String(path=w335) -> (string=w334:string)
                    n113 = Not Equal To 0?(x=w330) -> (x != 0?=w336:bool)
                    n114 = String Length(string=w334) -> (length=w333:i32)
                    n115 = Greater?(x=w333, y=5) -> (0:w329:bool)
                    n116 = Compound Arithmetic op=AND(w331, w336, w329) -> (w338:bool)
                    n117 = case shown="False" w338 {
                      tunnel: w342 -> [w344 w362]
                      tunnel: [w344 w361] -> w341
                      tunnel: w337 -> [_ w359]
                      tunnel: w340 -> [_ w358]
                      tunnel: [timestamp(0 s since 1904-01-01) ("*(type *) &x") w347] -> w339
                      tunnel: w335 -> [_ w346]
                      tunnel: w330 -> [_ w345]
                      frame False {
                        # "This cell wasn't active"
                      }
                      frame True {
                        w352 = sgl 3600.0  # To secs
                        w364 = TRUE  # ErrMsgOff
                        # "gets last elapsed time in hrs, adds to\nStart Time to get last clock time"
                        # "Reads the cell's data file"
                        n118 = Strip Path(path=w346) -> (stripped path=w366:path, name=w365:string)
                        n119 = call "Read Header and Spreadsheet File.vi"("DirIn"=w366, "NameIn"=w365, "ErrMsgOff"=w364) -> ("2D Data"=w354:sgl[][], "Error Out"=w363:errorcluster)  [unwired: 10 in, 5 out]
                        n120 = Unbundle By Name(w363) -> ("status"=w360:bool)
                        n121 = case shown="False" w360 {
                          tunnel: w362 -> [w372 w373]
                          tunnel: [w371 w373] -> w361
                          tunnel: w359 -> [w370 _]
                          tunnel: w354 -> [w369 _]
                          tunnel: w358 -> [w368 _]
                          frame False {
                            n122 = Bundle By Name(cluster=w370, "CurData"=w369) -> (w367:T7)
                            n123 = Replace Array Subset(array=w372, new element=w367, index=w368) -> (w371:T6)
                          }
                          frame True {
                            # "Error"
                          }
                        }
                        n124 = Index Array(array=w354, index (col)=0 ("disabled index (col)")) -> (element=w356:sgl[])  [unwired: 1 in]
                        n125 = Array Size(array=w356) -> (size(s)=w355:i32)
                        n126 = Decrement(x=w355) -> (x-1=w350:i32)
                        n127 = Index Array(array=w354, index (row)=w350, index (col)=0 ("index (row)")) -> (element=w353:sgl)
                        n128 = Multiply(x=w352, y=w353) -> (x*y=w351:sgl)
                        n129 = Add(x=w351, y=w345) -> (x+y=w348:dbl)
                        n130 = To Time Stamp(1:w348) -> (0:w347:timestamp)
                      }
                    }
                  }
                }
                frame #2 {
                  # "Final values"
                  n131 = Bundle By Name(cluster=w376, "Cell Data"=w375) -> (w374:T5)
                  n132 = global write "Global ER2007.vi" "Test Info"(w374) -> ()
                }
              }
            }
          }
          n133 = local write "Radio Cell Selects"("Radio Cell Selects") -> ()
          n134 = case shown="\"No Selection\"" "Radio Cell Selects" {
            tunnel: [u8 2 ("Disabled") u8 0 ("Disabled")] -> w179
            frame "No Selection" {
            }
            frame "CS 1", Default {
            }
          }
          n135 = property on="TakePt" class="Bool"("Disabled"=w179) -> ()  [unwired: 2 in, 2 out]
          n136 = property on="Setup" class="Bool"("Disabled"=w179) -> ()  [unwired: 2 in, 2 out]
          n137 = property on="History" class="Bool"("Disabled"=w179) -> ()  [unwired: 2 in, 2 out]
          n138 = local write "T-A (°C)"(w171) -> ()
          n139 = local write "Delta P (psi)"(w161) -> ()
          n140 = local write "ER 1-2"(w175) -> ()
          n141 = local write "ER 2-3"(w172) -> ()
          n142 = local write "T-B (°C)"(w170) -> ()
          n143 = local write "Pc-d(psig)"(w160) -> ()
          n144 = local write "Sample ID"(w176) -> ()
          n145 = local write "ER 1-3"(w174) -> ()
          n146 = local write "ER 1-4"(w173) -> ()
          n147 = local write "F 2-3"(w163) -> ()
          n148 = local write "NOP (psig)"(w169) -> ()
          n149 = local write "Pc (psig)"(w168) -> ()
          n150 = local write "Disp Pv (ml)"(w167) -> ()
          n151 = local write "Time"(w166) -> ()
          n152 = local write "Lapsed Hrs"(w165) -> ()
        }
        frame #8 {
          w381 = TRUE  # Init
          # "Other PC Idx"
          # "Inits the Sample Request vi"
          n153 = call "Sample Request Control.vi"("PC ID"=w380, "SimOn"=w383, "Init"=w381) -> ("ErrOut"=w382:errorcluster)  [unwired: 11 in, 5 out]
          n154 = case shown="1, Default" w380 {
            tunnel: [1 ("index") 0 ("index")] -> w379
            frame 1, Default {
            }
            frame 2 {
            }
          }
          n155 = call <vilib>:"Simple Error Handler.vi"("error in (no error)"=w382) -> ()  [unwired: 4 in, 5 out]
        }
        frame #9 {
          # "Starts the Background DAQ Task running"
          n156 = global read "Global ER2007.vi" "BckDaqLp vi name"() -> (w387:path)
          n157 = Array Size(array=w391) -> (size(s)=w390:i32)
          n158 = global read "Global ER2007.vi" "DAQ Run"() -> (w386:bool)
          n159 = Initialize Array(FALSE, w390) -> (w388:bool[])
          n160 = case shown="False" w386 {
            tunnel: w387 -> [w392 w399]
            frame False {
              # "Not running - start it up"
              n161 = stacked-sequence {
                tunnel: w392 -> [_ w394]
                frame #0 {
                  # "Set the Init flag"
                  n162 = global write "Global ER2007.vi" "DAQ Init"(TRUE ("A/D Init")) -> ()
                }
                frame #1 {
                  # "Run it"
                  n163 = Open VI Reference(vi path=w394) -> (vi reference=w398:refnum<vi>)  [unwired: 5 in, 1 out]
                  n164 = invoke class="VI" method="Run VI"(reference=w398, "Wait until done"=FALSE, "Auto Dispose Ref"=TRUE) -> (error out=w395:errorcluster)  [unwired: 2 in, 4 out]
                  n165 = call <vilib>:"Simple Error Handler.vi"("error in (no error)"=w395) -> ()  [unwired: 4 in, 5 out]
                }
              }
            }
            frame True {
              # "The bckgnd task is already running - stop it and restart"
              n166 = stacked-sequence {
                tunnel: w399 -> [_ _ _ w403]
                frame #0 {
                  # "Stop the task"
                  n167 = global write "Global ER2007.vi" "DAQ Stop"(TRUE ("A/D Stop")) -> ()
                }
                frame #1 {
                  # "Small wait"
                  n168 = Wait (ms)(milliseconds to wait=u32 500) -> ()  [unwired: 1 out]
                }
                frame #2 {
                  # "Set the Init flag"
                  n169 = global write "Global ER2007.vi" "DAQ Init"(TRUE ("A/D Init")) -> ()
                }
                frame #3 {
                  # "Restart the task"
                  n170 = Open VI Reference(vi path=w403) -> (vi reference=w407:refnum<vi>)  [unwired: 5 in, 1 out]
                  n171 = invoke class="VI" method="Run VI"(reference=w407, "Wait until done"=FALSE, "Auto Dispose Ref"=TRUE) -> (error out=w404:errorcluster)  [unwired: 2 in, 4 out]
                  n172 = call <vilib>:"Simple Error Handler.vi"("error in (no error)"=w404) -> ()  [unwired: 4 in, 5 out]
                }
              }
            }
          }
        }
        frame #10 {
          # "Starts the Get Cell Data background task"
          n173 = global read "Global ER2007.vi" "BckGetEng vi name"() -> (w408:path)
          n174 = stacked-sequence {
            tunnel: w408 -> [_ _ w412]
            frame #0 {
              w409 = FALSE ("GCD Go")
              # "Clears flags"
              n175 = global write "Global ER2007.vi" "GCD Go"(w409) -> ()
              n176 = global write "Global ER2007.vi" "GCD Err"(w409) -> ()
              n177 = global write "Global ER2007.vi" "GCD Busy"(w409) -> ()
              n178 = global write "Global ER2007.vi" "GCD Stop"(w409) -> ()
            }
            frame #1 {
              # "Small wait"
              n179 = Wait (ms)(milliseconds to wait=u32 500) -> ()  [unwired: 1 out]
            }
            frame #2 {
              # "If task is running, stop it; otherwise just start it"
              n180 = global read "Global ER2007.vi" "GCD Run"() -> (w411:bool)
              n181 = case shown="False" w411 {
                tunnel: w412 -> [w413 w419]
                frame False {
                  n182 = stacked-sequence {
                    tunnel: w413 -> [w414]
                    frame #0 {
                      n183 = Open VI Reference(vi path=w414) -> (vi reference=w415:refnum<vi>)  [unwired: 5 in, 1 out]
                      n184 = invoke class="VI" method="Run VI"(reference=w415, "Wait until done"=FALSE, "Auto Dispose Ref"=TRUE) -> (error out=w418:errorcluster)  [unwired: 2 in, 4 out]
                      n185 = call <vilib>:"Simple Error Handler.vi"("error in (no error)"=w418) -> ()  [unwired: 4 in, 5 out]
                    }
                  }
                }
                frame True {
                  # "task is still running"
                  n186 = stacked-sequence {
                    tunnel: w419 -> [_ _ _ _ w435]
                    frame #0 {
                      # "stops task"
                      n187 = global write "Global ER2007.vi" "GCD Stop"(TRUE ("GCD Stop")) -> ()
                    }
                    frame #1 {
                      # "Small wait"
                      n188 = Wait (ms)(milliseconds to wait=u32 500) -> ()  [unwired: 1 out]
                    }
                    frame #2 {
                      # "Waits for task to stop or timeout"
                      n189 = Get Date/Time In Seconds() -> (seconds since 1Jan1904=w423:timestamp)
                      n190 = To Double Precision Float(number=w423) -> (double precision float=w422:dbl)
                      n191 = while {
                        tunnel: w422 -> [w431]
                        stop <- w426 stop-if-true
                        n192 = Get Date/Time In Seconds() -> (seconds since 1Jan1904=w433:timestamp)
                        n193 = global read "Global ER2007.vi" "GCD Stop"() -> (w424:bool)
                        n194 = To Double Precision Float(number=w433) -> (double precision float=w432:dbl)
                        n195 = Wait Until Next ms Multiple(millisecond multiple=u32 250) -> ()  [unwired: 1 out]
                        n196 = Subtract(x=w432, y=w431) -> (x-y=w430:dbl)
                        n197 = Greater?(x=w430, y=8.0) -> (0:w427:bool)
                        n198 = Not(x=w424) -> (.not. x?=w425:bool)
                        n199 = Or(x=w427, y=w425) -> (x .or. y?=w426:bool)
                      }
                    }
                    frame #3 {
                      # "Small wait"
                      n200 = Wait (ms)(milliseconds to wait=u32 500) -> ()  [unwired: 1 out]
                    }
                    frame #4 {
                      # "Run it"
                      n201 = Open VI Reference(vi path=w435) -> (vi reference=w439:refnum<vi>)  [unwired: 5 in, 1 out]
                      n202 = invoke class="VI" method="Run VI"(reference=w439, "Wait until done"=FALSE, "Auto Dispose Ref"=TRUE) -> (error out=w436:errorcluster)  [unwired: 2 in, 4 out]
                      n203 = call <vilib>:"Simple Error Handler.vi"("error in (no error)"=w436) -> ()  [unwired: 4 in, 5 out]
                    }
                  }
                }
              }
            }
          }
        }
      }
    }
    frame #1 {
      # "Main\nloop"
      n204 = while {
        shift-right: [w475] -> _
        shift-left: w451 -> [w468]
        shift-right: [w476] -> _
        shift-left: w450 -> [w477]
        shift-right: [FALSE ("Init")] -> _
        shift-left: w449 -> [w474]
        shift-right: [w472] -> _
        shift-left: w448 -> [w471]
        shift-right: [w469] -> _
        shift-left: w447 -> [w470]
        shift-right: [w465] -> _
        shift-left: w445 -> [w466]
        shift-right: [w467] -> _
        shift-left: w446 -> [w464]
        shift-right: [w463] -> _
        shift-left: w444 -> [w462]
        shift-right: [w460] -> _
        shift-left: w443 -> [w461]
        tunnel: w442 -> [w455]
        tunnel: w441 -> [w454]
        shift-right: [w453] -> _
        shift-left: w440 -> [w452]
        stop <- w478 stop-if-true
        # "Stop IP"
        # "Refresh"
        # "Other PC Idx"
        # "Init"
        # "SimDAQ"
        # "CurSUPCell"
        # "CurGCDCell"
        # "CurSelectedCell"
        # "RadioSelect"
        # "TakePtActive"
        # "CurActiveCells"
        n205 = global read "Global ER2007.vi" "New Data"() -> (w459:bool)
        n206 = global read "Global ER2007.vi" "New Setup"() -> (w458:bool)
        n207 = global read "Global ER2007.vi" "GCD Prog"() -> (→"GCD Prog":bool[])
        n208 = global read "Global ER2007.vi" "TakePt"() -> (w457:bool)
        n209 = Wait Until Next ms Multiple(millisecond multiple=u32 333) -> ()  [unwired: 1 out]
        n210 = event shown="[0] Timeout" {
          selector: _ -> [_ _ _ _ _ _ _ _ _]
          dyn-events: _ -> [_ _ _ _ _ _ _ _ _]
          timeout: 333 -> [_ _ _ _ _ _ _ _ _]
          tunnel: [w499 w1169 w1188 w1215 w1243 w1278 w1289 w1308 w1319] -> w475
          tunnel: w468 -> [w500 w1169 w1188 w1215 w1243 w1278 w1289 w1308 w1319]
          tunnel: [w483 FALSE FALSE FALSE FALSE FALSE FALSE FALSE FALSE] -> w478
          tunnel: w477 -> [w487 _ w1187 w1214 w1242 w1279 w1288 w1309 w1320]
          tunnel: [w487 w1167 w1187 w1214 w1242 w1279 w1288 w1309 w1320] -> w476
          tunnel: w457 -> [w502 _ _ _ _ _ _ _ _]
          tunnel: w458 -> [w505 _ _ _ _ _ _ _ _]
          tunnel: w459 -> [w503 _ _ _ _ _ _ _ _]
          tunnel: w474 -> [w501 _ _ _ _ _ _ _ _]
          tunnel: [w498 w1168 w1186 w1213 w1241 w1268 w1287 w1307 w1318] -> w472
          tunnel: w471 -> [w497 w1168 w1186 w1213 w1241 w1268 w1287 w1307 w1318]
          tunnel: w470 -> [w485 w1166 w1185 w1212 w1240 w1267 w1286 w1306 w1317]
          tunnel: [w496 w1166 w1185 w1212 w1240 w1267 w1286 w1306 w1317] -> w469
          tunnel: w464 -> [w493 w1165 w1184 w1211 w1239 w1265 w1284 w1303 w1315]
          tunnel: [w494 w1165 w1184 w1211 w1239 w1265 w1284 w1303 w1315] -> w467
          tunnel: w466 -> [w492 w1164 w1183 w1209 w1238 w1266 w1285 w1305 w1316]
          tunnel: [w495 w1163 w1183 w1209 w1238 w1266 w1285 w1305 w1316] -> w465
          tunnel: [w490 w1162 w1182 w1210 w1237 w1264 w1283 w1304 w1314] -> w463
          tunnel: w462 -> [w491 w1162 w1182 _ w1237 w1264 w1283 w1304 w1314]
          tunnel: w461 -> [w489 _ w1181 w1208 w1236 w1263 w1282 w1302 w1313]
          tunnel: [w488 TRUE w1181 w1208 w1236 w1263 w1282 w1302 w1313] -> w460
          tunnel: w455 -> [w486 _ _ _ _ _ _ _ _]
          tunnel: w454 -> [w484 _ _ _ _ _ _ _ _]
          tunnel: [w481 w1160 w1180 w1207 w1235 w1262 w1281 w1300 TRUE] -> w453
          tunnel: w452 -> [w482 w1160 w1180 w1207 w1235 w1262 w1281 w1300 _]
          event Timeout {
            # "Timeout"
            n211 = event-data() -> ()  [unwired: 1 in, 1 out]
            n212 = Compound Arithmetic op=OR(w503, w505, w502, w501) -> (w504:bool)
            n213 = case shown="True" w504 {
              tunnel: w503 -> [_ w825]
              tunnel: w502 -> [_ w824]
              tunnel: w500 -> [w522 w807]
              tunnel: [w521 w806] -> w499
              tunnel: [w523 w811] -> w498
              tunnel: w497 -> [w523 w810]
              tunnel: w485 -> [w520 w809]
              tunnel: [w519 w808] -> w496
              tunnel: w492 -> [w518 w802]
              tunnel: [w517 w802] -> w495
              tunnel: [w516 w805] -> w494
              tunnel: w493 -> [w515 w805]
              tunnel: w491 -> [w514 w803]
              tunnel: [w513 w804] -> w490
              tunnel: w489 -> [w512 _]
              tunnel: [w511 w801] -> w488
              tunnel: w486 -> [w510 _]
              tunnel: w484 -> [w509 _]
              tunnel: [w508 FALSE] -> w483
              tunnel: w482 -> [w507 w796]
              tunnel: [w506 w796] -> w481
              frame False {
                n214 = stacked-sequence {
                  seq-local: [w535 _ _] -> [_ w622 _]
                  seq-local: [w530 _ _] -> [_ w621 _]
                  seq-local: [w546 _ _] -> [_ w618 _]
                  seq-local: [w542 _ _] -> [_ w613 _]
                  tunnel: w523 -> [w552 _ _]
                  tunnel: w522 -> [w551 w620 _]
                  tunnel: [_ w619 _] -> w521
                  tunnel: w520 -> [w550 w611 _]
                  tunnel: [_ w612 _] -> w519
                  tunnel: w518 -> [_ w615 w751]
                  tunnel: [_ _ w751] -> w517
                  tunnel: [_ w617 _] -> w516
                  tunnel: w515 -> [w547 w614 _]
                  tunnel: w514 -> [w545 _ w750]
                  tunnel: [_ _ w749] -> w513
                  tunnel: w512 -> [w541 _ _]
                  tunnel: [_ w616 _] -> w511
                  tunnel: w510 -> [w532 _ _]
                  tunnel: w509 -> [w529 _ _]
                  tunnel: [_ _ w743] -> w508
                  tunnel: w507 -> [_ _ w745]
                  tunnel: [_ _ w744] -> w506
                  frame #0 {
                    # "TRUE if time to sample a cell"
                    # "Sample cell index"
                    # "Checks if sample req'd"
                    n215 = local read "GCD Busy"() -> (w543:bool)
                    n216 = global read "Global ER2007.vi" "GCD Busy"() -> (w538:bool)
                    n217 = Get Date/Time In Seconds() -> (seconds since 1Jan1904=w549:timestamp)
                    n218 = global read "Global ER2007.vi" "GCD Err"() -> (→"GCD Err":bool)
                    n219 = To Double Precision Float(number=w549) -> (double precision float=w548:dbl)
                    "Cur Time" <- w548
                    n220 = Not Equal?(x=w543, y=w538) -> (x != y?=w544:bool)
                    n221 = case shown="False" w538 {
                      tunnel: w552 -> [w565 _]
                      tunnel: w551 -> [w575 _]
                      tunnel: [w574 0] -> w530
                      tunnel: [w573 w609] -> w534
                      tunnel: w550 -> [w572 _]
                      tunnel: w548 -> [w570 _]
                      tunnel: w545 -> [w568 _]
                      frame False {
                        n222 = case shown="0, Default" w568 {
                          tunnel: [-1 0 1 2 3 4] -> w569
                          frame 0, Default {
                          }
                          frame 1 {
                          }
                          frame 2 {
                          }
                          frame 3 {
                          }
                          frame 4 {
                          }
                          frame 5 {
                          }
                        }
                        n223 = Array Size(array=w565) -> (size(s)=w567:i32)
                        n224 = Or Array Elements(Boolean array=w572) -> (logical OR=w571:bool)
                        n225 = Decrement(x=w567) -> (x-1=w566:i32)
                        n226 = case shown="False" w571 {
                          tunnel: w565 -> [w588 _]
                          tunnel: w575 -> [w587 _]
                          tunnel: [w586 w604] -> w574
                          tunnel: [w585 w605] -> w573
                          tunnel: w572 -> [_ w606]
                          tunnel: w570 -> [w584 _]
                          tunnel: w569 -> [w583 _]
                          tunnel: w566 -> [w582 _]
                          frame False {
                            # "Normal sample checker"
                            n227 = while {
                              tunnel: w588 -> [w599] mode=indexing
                              tunnel: w582 -> [w598]
                              tunnel: w587 -> [w597] mode=indexing
                              tunnel: w584 -> [w596]
                              tunnel: [w592] -> w586
                              tunnel: [w595] -> w585
                              tunnel: w583 -> [w593]
                              i -> [w592]
                              stop <- w591 stop-if-true
                              # "NOT current SUP cell"
                              n228 = case shown="True" w599 {
                                tunnel: w597 -> [_ w602]
                                tunnel: w596 -> [_ w603]
                                tunnel: [FALSE w601] -> w595
                                frame False {
                                # "Not Active"
                                }
                                frame True {
                                # "This cell is active - see\nif is time for a sample"
                                n229 = Less Or Equal?(x=w602, y=w603) -> (x <= y?=w601:bool)
                                }
                              }
                              n230 = Not Equal?(x=w592, y=w593) -> (x != y?=w589:bool)
                              n231 = Less Or Equal?(x=w598, y=w592) -> (x <= y?=w594:bool)
                              n232 = Or(x=w595, y=w594) -> (x .or. y?=w590:bool)
                              n233 = And(x=w590, y=w589) -> (x .and. y?=w591:bool)
                            }
                          }
                          frame True {
                            w605 = TRUE  # Take Pt Sample
                            # "TakePt is active"
                            n234 = while {
                              tunnel: w606 -> [w607] mode=indexing
                              tunnel: [w608] -> w604
                              i -> [w608]
                              stop <- w607 stop-if-true
                            }
                          }
                        }
                      }
                      frame True {
                        w609 = FALSE  # Don't sample
                        # "\"Get Cell Data.vi\" is still busy"
                      }
                    }
                    n235 = case shown="True" w544 {
                      tunnel: w547 -> [w558 w562]
                      tunnel: [w558 w561] -> w546
                      tunnel: w538 -> [_ w560]
                      tunnel: [w557 TRUE] -> w542
                      tunnel: w541 -> [w557 _]
                      frame False {
                      }
                      frame True {
                        n236 = case shown="False" w560 {
                          tunnel: w562 -> [_ w564]
                          tunnel: [w563 w564] -> w561
                          frame False {
                            w563 = 0  # <none>
                          }
                          frame True {
                          }
                        }
                        "GCD Busy" <- w560
                      }
                    }
                    n237 = global read "Global ER2007.vi" "DAQ Run"() -> (→"DAQ Run":bool)
                    n238 = local read "System Error"() -> (w539:bool)
                    n239 = global read "Global ER2007.vi" "A/D Err"() -> (w525:bool)
                    n240 = global read "Global ER2007.vi" "Galil Err"() -> (w526:bool)
                    n241 = Or(x=w525, y=w526) -> (x .or. y?=w524:bool)
                    n242 = Not Equal?(x=w539, y=w524) -> (x != y?=w540:bool)
                    n243 = case shown="True" w540 {
                      tunnel: w524 -> [_ w554]
                      tunnel: w526 -> [_ w555]
                      tunnel: w525 -> [_ w556]
                      frame False {
                      }
                      frame True {
                        n244 = property on="System Error" class="Bool (strict)"("Visible"=w554) -> ()  [unwired: 2 in, 2 out]
                        n245 = property on="Reset DAQ" class="Bool"("Visible"=w554) -> ()  [unwired: 2 in, 2 out]
                        "A/D Err" <- w556
                        "System Error" <- w554
                        "VPA Err" <- w555
                      }
                    }
                    n246 = global read "Global ER2007.vi" "GCD Reset"() -> (w531:bool)
                    "GCD Reset" <- w531
                    n247 = call "Sample Request Control.vi"("Sample Request"=w534, "SimOn"=w532, "Reset"=w531) -> ("Request Granted"=w535:bool, "Reset Done"=w533:bool, "Busy Status"=w527:bool[])  [unwired: 11 in, 3 out]
                    n248 = case shown="True" w533 {
                      frame False {
                      }
                      frame True {
                        n249 = global write "Global ER2007.vi" "GCD Reset"(FALSE ("GCD Reset")) -> ()
                      }
                    }
                    n250 = Index Array(array=w527, index=w529) -> (element=→"Other PC Busy":bool)
                    n251 = global write "Global ER2007.vi" "BoxBusy"(w527) -> ()
                  }
                  frame #1 {
                    n252 = case shown="True" w622 {
                      tunnel: w621 -> [_ w680]
                      tunnel: w620 -> [w628 w679]
                      tunnel: [w628 w678] -> w619
                      tunnel: [w625 w677] -> w617
                      tunnel: w618 -> [w625 _]
                      tunnel: [w627 TRUE] -> w616
                      tunnel: w615 -> [w626 _]
                      tunnel: w614 -> [_ _]
                      tunnel: w613 -> [w624 _]
                      tunnel: [w623 w675] -> w612
                      tunnel: w611 -> [w623 w674]
                      frame False {
                        # "No sample req'd or possible at this time"
                        n253 = case shown="True" w624 {
                          tunnel: [FALSE FALSE] -> w627
                          tunnel: w626 -> [_ w636]
                          tunnel: w625 -> [_ w631]
                          tunnel: w623 -> [_ w630]
                          frame False {
                          }
                          frame True {
                            # "Update control visible properties"
                            n254 = case shown="1, Default" w636 {
                              selector: w636 -> [_ w648]
                              tunnel: [u8 2 ("Disabled") w650] -> w635
                              tunnel: [u8 2 ("Disabled") w642] -> w634
                              tunnel: [u8 2 ("Disabled") w655] -> w633
                              tunnel: [u8 0 ("Disabled") u8 0 ("Disabled")] -> w632
                              tunnel: w631 -> [_ w652]
                              tunnel: w630 -> [_ w646]
                              frame 0 {
                              }
                              frame 1, Default {
                                w643 = u8 2 ("Disabled")
                                # "TRUE if Radio button = CurGCDCell"
                                n255 = global read "Global ER2007.vi" "Test Info"() -> (w649:T5)
                                n256 = Or Array Elements(Boolean array=w646) -> (logical OR=w645:bool)
                                n257 = Decrement(x=w648) -> (x-1=w647:i32)
                                n258 = Equal?(x=w648, y=w652) -> (x = y?=w651:bool)
                                n259 = Unbundle By Name(w649) -> ("Cell Data"=w653:T6)
                                n260 = Index Array(array=w653, index=w647) -> (element=w673:T7)
                                n261 = Unbundle By Name(w673) -> ("Length"=w672:dbl, "Diameter"=w670:dbl, "ElectSpace"=w671:dbl, "CurData"=w663:dbl[][])
                                n262 = Less Or Equal To 0?(x=w671) -> (x <= 0?=w667:bool)
                                n263 = Less Or Equal To 0?(x=w672) -> (x <= 0?=w669:bool)
                                n264 = Index Array(array=w663, index (col)=0 ("disabled index (col)")) -> (element=w662:dbl[])  [unwired: 1 in]
                                n265 = Less Or Equal To 0?(x=w670) -> (x <= 0?=w668:bool)
                                n266 = Array Size(array=w662) -> (size(s)=w661:i32)
                                n267 = Select(t=u8 2 ("Disabled"), s=w651, f=u8 0) -> (s? t:f=w650:u8)
                                n268 = Compound Arithmetic op=OR(w669, w668, w667) -> (w666:bool)
                                n269 = Less?(x=w661, y=2) -> (x < y?=w660:bool)
                                n270 = Select(t=w643, s=w666, f=w650) -> (s? t:f=w644:u8)
                                n271 = Select(t=u8 2 ("Disabled"), s=w660, f=u8 0 ("Disabled")) -> (s? t:f=w655:u8)
                                n272 = Select(t=w643, s=w645, f=w644) -> (s? t:f=w642:u8)
                              }
                            }
                            n273 = property on="Setup" class="Bool"("Disabled"=w635) -> ()  [unwired: 2 in, 2 out]
                            n274 = property on="TakePt" class="Bool"("Disabled"=w634) -> ()  [unwired: 2 in, 2 out]
                            n275 = property on="History" class="Bool"("Disabled"=w633) -> ()  [unwired: 2 in, 2 out]
                            n276 = property on="CurVals" class="Bool"("Disabled"=w632) -> ()  [unwired: 2 in, 2 out]
                          }
                        }
                      }
                      frame True {
                        # "Sample\nreq'd"
                        n277 = stacked-sequence {
                          tunnel: w680 -> [w683 w707]
                          tunnel: w679 -> [w695 _]
                          tunnel: [w694 _] -> w678
                          tunnel: [w687 _] -> w677
                          tunnel: [w686 _] -> w675
                          tunnel: w674 -> [w685 _]
                          frame #0 {
                            # "Updates Next\nTime, sets flags"
                            n278 = global read "Global ER2007.vi" "Test Info"() -> (w690:T5)
                            n279 = Boolean To (0,1)(Boolean=w685) -> (0, 1=w684:i16[])
                            n280 = Unbundle By Name(w690) -> ("Cell Data"=w698:T6)
                            n281 = Index Array(array=w684, index=w683) -> (element=w682:i16)
                            n282 = Index Array(array=w698, index=w683) -> (element=w699:T7)
                            n283 = Greater Than 0?(x=w682) -> (x > 0?=w681:bool)
                            n284 = global write "Global ER2007.vi" "GCD Busy"(TRUE ("GCD Busy")) -> ()
                            n285 = Unbundle By Name(w699) -> ("Cell ID"=w687:i32, "DAQ Period"=w701:u32, "DAQ Units"=w700:u16, "Start Time"=w692:dbl, "Next Time"=w693:dbl)
                            "Selected Data Cell" <- w687
                            n286 = case shown="True" w681 {
                              tunnel: [w702 w704] -> w686
                              tunnel: w685 -> [w702 w703]
                              frame False {
                              }
                              frame True {
                                n287 = Array Size(array=w703) -> (size(s)=w706:i32)
                                n288 = Initialize Array(FALSE, w706) -> (w704:bool[])
                              }
                            }
                            n289 = call "Sample Timer Functions.vi"("Next Time In"=w693, "Start Time"=w692, "DAQ Units"=w700, "DAQ Period"=w701) -> ("New Time Out"=w691:dbl)  [unwired: 2 in, 5 out]
                            n290 = Replace Array Subset(array=w695, new element=w691, index=w683) -> (w694:dbl[])
                            n291 = Bundle By Name(cluster=w699, "Next Time"=w691) -> (w696:T7)
                            n292 = Replace Array Subset(array=w698, new element=w696, index=w683) -> (w697:T6)
                            n293 = Bundle By Name(cluster=w690, "CurCell"=w687, "Cell Data"=w697) -> (w689:T5)
                            n294 = global write "Global ER2007.vi" "Test Info"(w689) -> ()
                            n295 = global write "Global ER2007.vi" "DataCell"(w687) -> ()
                            "Cell Data Idx" <- w683
                          }
                          frame #1 {
                            w710 = cluster{u32, u32}[] [{1985280, 1985280}, {6618880, 6618880}, {1985280, 1985280}, {6618880, 6618880}]  # Busy Colors
                            # "Runs the \"Get Cell Data.vi\"; lights the\n\"Busy\" LED"
                            n296 = global read "Global ER2007.vi" "GCD Run"() -> (w708:bool)
                            n297 = case shown="False" w708 {
                              frame False {
                                # "NOT running for some reason"
                                n298 = stacked-sequence {
                                seq-local: [w712 _ _] -> [_ w719 _]
                                seq-local: [_ w718 _] -> [_ _ w729]
                                frame #0 {
                                n299 = global read "Global ER2007.vi" "BckGetEng vi name"() -> (w711:path)
                                n300 = Get Date/Time In Seconds() -> (seconds since 1Jan1904=w713:timestamp)
                                n301 = To Double Precision Float(number=w713) -> (double precision float=w712:dbl)
                                n302 = Open VI Reference(vi path=w711) -> (vi reference=w714:refnum<vi>)  [unwired: 5 in, 1 out]
                                n303 = invoke class="VI" method="Run VI"(reference=w714, "Wait until done"=FALSE, "Auto Dispose Ref"=TRUE) -> (error out=w717:errorcluster)  [unwired: 2 in, 4 out]
                                n304 = call <vilib>:"Simple Error Handler.vi"("error in (no error)"=w717) -> ()  [unwired: 4 in, 5 out]
                                }
                                frame #1 {
                                n305 = while {
                                tunnel: w719 -> [w726]
                                tunnel: [w721] -> w718
                                stop <- w722 stop-if-true
                                # "Waits for Run flag or T/O"
                                n306 = Get Date/Time In Seconds() -> (seconds since 1Jan1904=w728:timestamp)
                                n307 = To Double Precision Float(number=w728) -> (double precision float=w727:dbl)
                                n308 = global read "Global ER2007.vi" "GCD Run"() -> (w720:bool)
                                n309 = Wait Until Next ms Multiple(millisecond multiple=u32 250) -> ()  [unwired: 1 out]
                                n310 = Subtract(x=w727, y=w726) -> (x-y=w725:dbl)
                                n311 = Greater?(x=w725, y=2.0) -> (0:w721:bool)
                                n312 = Or(x=w721, y=w720) -> (x .or. y?=w722:bool)
                                }
                                }
                                frame #2 {
                                n313 = case shown="False" w729 {
                                frame False {
                                # "Get cell data"
                                n314 = global write "Global ER2007.vi" "GCD Go"(TRUE ("GCD Run")) -> ()
                                }
                                frame True {
                                # "T/O error"
                                n315 = global write "Global ER2007.vi" "GCD Busy"(FALSE ("GCD Busy")) -> ()
                                }
                                }
                                }
                                }
                              }
                              frame True {
                                # "Get cell data"
                                n316 = global write "Global ER2007.vi" "GCD Go"(TRUE ("GCD Run")) -> ()
                              }
                            }
                            n317 = case shown="1" w707 {
                              tunnel: w710 -> [w734 w735 w737 w739 w741]
                              tunnel: TRUE ("C1-Status") -> [w733 w736 w738 w740 w742]
                              frame 0, Default {
                                n318 = property on="C1-Status" class="Bool (strict)"("Value"=w733, "Colors [4]"=w734) -> ()  [unwired: 2 in, 2 out]
                              }
                              frame 1 {
                                n319 = property on="C2-Status" class="Bool (strict)"("Value"=w736, "Colors [4]"=w735) -> ()  [unwired: 2 in, 2 out]
                              }
                              frame 2 {
                                n320 = property on="C3-Status" class="Bool (strict)"("Value"=w738, "Colors [4]"=w737) -> ()  [unwired: 2 in, 2 out]
                              }
                              frame 3 {
                                n321 = property on="C4-Status" class="Bool (strict)"("Value"=w740, "Colors [4]"=w739) -> ()  [unwired: 2 in, 2 out]
                              }
                              frame 4 {
                                n322 = property on="C5-Status" class="Bool (strict)"("Value"=w742, "Colors [4]"=w741) -> ()  [unwired: 2 in, 2 out]
                              }
                            }
                          }
                        }
                      }
                    }
                  }
                  frame #2 {
                    # "Updates the Cell Status; clears cur SUP cell;  grays out\nSetup button if active GCD cell and current selected cell\nare the same"
                    n323 = global read "Global ER2007.vi" "New GCD Status"() -> (w747:bool)
                    n324 = global read "Global ER2007.vi" "New Sup Status"() -> (w746:bool)
                    n325 = Or(x=w747, y=w746) -> (x .or. y?=w752:bool)
                    n326 = global read "Global ER2007.vi" "SUP Done"() -> (w748:bool)
                    n327 = case shown="True" w752 {
                      tunnel: w747 -> [_ w781]
                      tunnel: w746 -> [_ w780]
                      tunnel: w751 -> [_ _]
                      tunnel: w745 -> [w758 w779]
                      tunnel: [w757 w779] -> w744
                      tunnel: [w756 FALSE] -> w743
                      frame False {
                        # "Updates clock time"
                        n328 = case shown="True" w758 {
                          selector: w758 -> [w761 w763]
                          tunnel: [w761 w765] -> w757
                          tunnel: [FALSE w764] -> w756
                          frame False {
                          }
                          frame True {
                            # "STOP (Exit) in progress"
                            n329 = stacked-sequence {
                              seq-local: [w768 _] -> [_ w775]
                              tunnel: [w767 _] -> w765
                              tunnel: [_ w774] -> w764
                              tunnel: w763 -> [w766 _]
                              frame #0 {
                                n330 = global read "Global ER2007.vi" "STOP Done"() -> (w769:bool)
                                n331 = case shown="False" w769 {
                                tunnel: [FALSE ("STOP Ans") w773] -> w768
                                tunnel: [w770 FALSE] -> w767
                                tunnel: w766 -> [w770 _]
                                frame False {
                                }
                                frame True {
                                n332 = global read "Global ER2007.vi" "STOP Ans"() -> (w773:bool)
                                }
                                }
                              }
                              frame #1 {
                                n333 = case shown="False" w775 {
                                tunnel: [FALSE w777] -> w774
                                frame False {
                                }
                                frame True {
                                w777 = TRUE
                                n334 = global write "Global ER2007.vi" "DAQ Stop"(w777) -> ()
                                n335 = global write "Global ER2007.vi" "GCD Stop"(w777) -> ()
                                }
                                }
                              }
                            }
                          }
                        }
                        n336 = Get Date/Time String(want seconds? (F)=TRUE) -> (time string=→"Clock":string)  [unwired: 2 in, 1 out]
                      }
                      frame True {
                        # "Cell Status File needs to be updated"
                        n337 = stacked-sequence {
                          seq-local: [w783 _] -> [_ w794]
                          tunnel: w781 -> [w784 _]
                          tunnel: w780 -> [w782 _]
                          frame #0 {
                            # "Clear flags &\ngrab initial vals"
                            n338 = case shown="True" w784 {
                              tunnel: [w785 w790] -> w783
                              tunnel: w782 -> [w786 _]
                              frame False {
                                n339 = case shown="False" w786 {
                                tunnel: [w787 w788] -> w785
                                frame False {
                                w787 = 0  # <none>
                                }
                                frame True {
                                n340 = global read "Global ER2007.vi" "SupStatusCell"() -> (w788:i32)
                                n341 = global write "Global ER2007.vi" "New Sup Status"(FALSE ("New Status")) -> ()
                                }
                                }
                              }
                              frame True {
                                n342 = global read "Global ER2007.vi" "GCDStatusCell"() -> (w790:i32)
                                n343 = global write "Global ER2007.vi" "New GCD Status"(FALSE ("New GCD Status")) -> ()
                              }
                            }
                          }
                          frame #1 {
                            # "Updates Cell Status file"
                            n344 = global read "Global ER2007.vi" "Test Info"() -> (w792:T5)
                            n345 = global read "Global ER2007.vi" "Status File Path"() -> (w793:path)
                            n346 = call "Write Cell Status File.vi"("Cell Select"=w794, "Test Info"=w792, "Filepath"=w793) -> ()  [unwired: 8 in, 1 out]
                          }
                        }
                      }
                    }
                    n347 = case shown="True" w748 {
                      tunnel: w750 -> [w753 _]
                      tunnel: [w753 w754] -> w749
                      frame False {
                      }
                      frame True {
                        w754 = 0  # <none>
                        n348 = global write "Global ER2007.vi" "SUP Done"(FALSE ("SUP Done")) -> ()
                      }
                    }
                  }
                }
              }
              frame True {
                # "Something\nchanged"
                n349 = global read "Global ER2007.vi" "Test Info"() -> (w800:T5)
                n350 = case shown="True" w825 {
                  tunnel: w824 -> [w851 _]
                  tunnel: w800 -> [w831 w1028]
                  tunnel: [w850 w1043] -> w823
                  tunnel: [w849 w1042] -> w822
                  tunnel: [w848 w1041] -> w821
                  tunnel: [w847 w1040] -> w820
                  tunnel: [w846 w1039] -> w819
                  tunnel: [w845 w1038] -> w818
                  tunnel: [w844 w1037] -> w817
                  tunnel: [w843 w1036] -> w816
                  tunnel: [w842 w1035] -> w815
                  tunnel: [w841 w1034] -> w798
                  tunnel: [w840 w1033] -> w814
                  tunnel: [w839 w1032] -> w813
                  tunnel: [w838 w1031] -> w811
                  tunnel: [w837 w1030] -> w812
                  tunnel: w810 -> [w836 w1029]
                  tunnel: w809 -> [w835 w1027]
                  tunnel: [w834 w1027] -> w808
                  tunnel: w807 -> [w832 w1026]
                  tunnel: [w833 w1026] -> w806
                  tunnel: [w830 w1025] -> w804
                  tunnel: w803 -> [w829 w1025]
                  tunnel: [w828 w1024] -> w801
                  tunnel: [w827 w1023] -> w797
                  tunnel: [w826 w1022] -> w799
                  frame False {
                    n351 = case shown="False" w851 {
                      tunnel: [w874 w1015] -> w850
                      tunnel: [w857 w1014] -> w849
                      tunnel: [w858 w1013] -> w848
                      tunnel: [w859 w1012] -> w847
                      tunnel: [w860 w1011] -> w846
                      tunnel: [w862 w1010] -> w845
                      tunnel: [w863 w1009] -> w844
                      tunnel: [w864 w1008] -> w843
                      tunnel: [w865 w1007] -> w842
                      tunnel: [w866 w989] -> w841
                      tunnel: [w867 w1006] -> w840
                      tunnel: [w868 w1005] -> w839
                      tunnel: [w873 w1001] -> w838
                      tunnel: [w861 w1002] -> w837
                      tunnel: w836 -> [w872 w1001]
                      tunnel: w835 -> [w871 w999]
                      tunnel: [w871 w1000] -> w834
                      tunnel: [w869 w997] -> w833
                      tunnel: w832 -> [w870 w997]
                      tunnel: w831 -> [w856 w996]
                      tunnel: [w855 w995] -> w830
                      tunnel: w829 -> [_ w995]
                      tunnel: [w854 TRUE] -> w828
                      tunnel: [w853 w990] -> w827
                      tunnel: [w852 w988] -> w826
                      frame False {
                        n352 = stacked-sequence {
                          seq-local: [w881 _ _] -> [_ w903 _]
                          seq-local: [w880 _ _] -> [_ w906 _]
                          seq-local: [w879 _ _] -> [_ w905 _]
                          seq-local: [w876 _ _] -> [_ w904 _]
                          tunnel: [_ w936 _] -> w874
                          tunnel: [_ w934 _] -> w873
                          tunnel: w872 -> [_ w933 _]
                          tunnel: w870 -> [_ w932 _]
                          tunnel: [_ w931 _] -> w869
                          tunnel: [_ w919 _] -> w868
                          tunnel: [_ w918 _] -> w867
                          tunnel: [_ w917 _] -> w866
                          tunnel: [_ w916 _] -> w865
                          tunnel: [_ w915 _] -> w864
                          tunnel: [_ w914 _] -> w863
                          tunnel: [_ w913 _] -> w862
                          tunnel: [_ w912 _] -> w861
                          tunnel: [_ w911 _] -> w860
                          tunnel: [_ w910 _] -> w859
                          tunnel: [_ w909 _] -> w858
                          tunnel: [_ w908 _] -> w857
                          tunnel: w856 -> [w878 _ _]
                          tunnel: [_ _ w983] -> w855
                          tunnel: [_ _ TRUE] -> w854
                          tunnel: [_ w901 _] -> w853
                          tunnel: [_ w900 _] -> w852
                          frame #0 {
                            # "Updates Busy Captions"
                            # "New Setup"
                            n353 = global read "Global ER2007.vi" "SetupCell"() -> (w877:i32)
                            n354 = global read "Global ER2007.vi" "No Galil"() -> (w875:bool[])
                            n355 = Unbundle By Name(w878) -> ("Cell Data"=w883:T6)
                            n356 = Decrement(x=w877) -> (x-1=w876:i32)
                            n357 = for {
                              tunnel: w875 -> [w886] mode=indexing
                              i -> [w889]
                              n358 = Select(t="Manual", s=w886, f="VPA") -> (s? t:f=w885:string)
                              n359 = case shown="2" w889 {
                                tunnel: w885 -> [_ w890 w891 w892 w893 w894]
                                frame 0, Default {
                                }
                                frame 1 {
                                n360 = property on="C1-Status" class="Bool (strict)"("Caption.Text"=w890) -> ()  [unwired: 2 in, 2 out]
                                }
                                frame 2 {
                                n361 = property on="C2-Status" class="Bool (strict)"("Caption.Text"=w891) -> ()  [unwired: 2 in, 2 out]
                                }
                                frame 3 {
                                n362 = property on="C3-Status" class="Bool (strict)"("Caption.Text"=w892) -> ()  [unwired: 2 in, 2 out]
                                }
                                frame 4 {
                                n363 = property on="C4-Status" class="Bool (strict)"("Caption.Text"=w893) -> ()  [unwired: 2 in, 2 out]
                                }
                                frame 5 {
                                n364 = property on="C5-Status" class="Bool (strict)"("Caption.Text"=w894) -> ()  [unwired: 2 in, 2 out]
                                }
                              }
                            }
                            n365 = Index Array(array=w883, index=w876) -> (element=w884:T7)
                            n366 = Unbundle By Name(w884) -> ("Next Time"=w881:dbl, "Sample #"=w880:string, "Cell Status"=w882:enum16{"Inactive", "Setup", "Active", "Done"})
                            n367 = case shown="\"Active\"" w882 {
                              tunnel: [FALSE TRUE] -> w879
                              frame "Inactive", Default {
                              }
                              frame "Active" {
                              }
                            }
                          }
                          frame #1 {
                            # "New Setup"
                            n368 = local read "Sample ID"() -> (w935:string[])
                            n369 = global read "Global ER2007.vi" "SUP Cleared"() -> (w902:bool)
                            n370 = case shown="True" w902 {
                              frame False {
                              }
                              frame True {
                                n371 = global write "Global ER2007.vi" "SUP Cleared"(FALSE ("SUP Cleared")) -> ()
                              }
                            }
                            n372 = Replace Array Subset(array=w933, new element=w905, index=w904) -> (w934:bool[])
                            n373 = Replace Array Subset(array=w935, new element=w906, index=w904) -> (w936:string[])
                            n374 = local read "Delta P (psi)"() -> (w898:dbl[])
                            n375 = local read "Disp Pv (ml)"() -> (w899:dbl[])
                            n376 = local read "Lapsed Hrs"() -> (w920:dbl[])
                            n377 = local read "NOP (psig)"() -> (w923:dbl[])
                            n378 = local read "Pc-d(psig)"() -> (w897:dbl[])
                            n379 = local read "Pc (psig)"() -> (w922:dbl[])
                            n380 = local read "T-A (°C)"() -> (w925:dbl[])
                            n381 = local read "T-B (°C)"() -> (w924:dbl[])
                            n382 = local read "ER 1-2"() -> (w930:dbl[])
                            n383 = local read "ER 2-3"() -> (w927:dbl[])
                            n384 = local read "ER 1-3"() -> (w929:dbl[])
                            n385 = local read "ER 1-4"() -> (w928:dbl[])
                            n386 = Replace Array Subset(array=w932, new element=w903, index=w904) -> (w931:dbl[])
                            n387 = local read "F 2-3"() -> (w926:dbl[])
                            n388 = local read "Time"() -> (w921:timestamp[])
                            n389 = case shown="False" w902 {
                              tunnel: w930 -> [w951 w981]
                              tunnel: w929 -> [w950 w976]
                              tunnel: w928 -> [w949 w975]
                              tunnel: w927 -> [w948 w974]
                              tunnel: w926 -> [w947 w973]
                              tunnel: w925 -> [w946 w965]
                              tunnel: w924 -> [w945 w964]
                              tunnel: w923 -> [w944 w963]
                              tunnel: w922 -> [w943 w962]
                              tunnel: w898 -> [w942 w961]
                              tunnel: w921 -> [w941 w960]
                              tunnel: w920 -> [w940 w959]
                              tunnel: [w940 w972] -> w919
                              tunnel: [w941 w971] -> w918
                              tunnel: [w942 w970] -> w917
                              tunnel: [w943 w969] -> w916
                              tunnel: [w944 w968] -> w915
                              tunnel: [w945 w967] -> w914
                              tunnel: [w946 w966] -> w913
                              tunnel: [w947 w977] -> w912
                              tunnel: [w948 w978] -> w911
                              tunnel: [w949 w979] -> w910
                              tunnel: [w950 w980] -> w909
                              tunnel: [w951 w982] -> w908
                              tunnel: w904 -> [_ w952]
                              tunnel: timestamp(0 s since 1904-01-01) ("*(type *) &x") -> [_ w958]
                              tunnel: [w939 w957] -> w901
                              tunnel: w897 -> [w939 w956]
                              tunnel: [w938 w953] -> w900
                              tunnel: w899 -> [w938 w954]
                              frame False {
                              }
                              frame True {
                                w955 = 0.0 ("new element/subarray")
                                n390 = Replace Array Subset(array=w961, new element=w955, index=w952) -> (w970:dbl[])
                                n391 = Replace Array Subset(array=w959, new element=w955, index=w952) -> (w972:dbl[])
                                n392 = Replace Array Subset(array=w954, new element=w955, index=w952) -> (w953:dbl[])
                                n393 = Replace Array Subset(array=w976, new element=w955, index=w952) -> (w980:dbl[])
                                n394 = Replace Array Subset(array=w974, new element=w955, index=w952) -> (w978:dbl[])
                                n395 = Replace Array Subset(array=w965, new element=w955, index=w952) -> (w966:dbl[])
                                n396 = Replace Array Subset(array=w963, new element=w955, index=w952) -> (w968:dbl[])
                                n397 = Replace Array Subset(array=w960, new element=w958, index=w952) -> (w971:timestamp[])
                                n398 = Replace Array Subset(array=w981, new element=w955, index=w952) -> (w982:dbl[])
                                n399 = Replace Array Subset(array=w975, new element=w955, index=w952) -> (w979:dbl[])
                                n400 = Replace Array Subset(array=w973, new element=w955, index=w952) -> (w977:dbl[])
                                n401 = Replace Array Subset(array=w964, new element=w955, index=w952) -> (w967:dbl[])
                                n402 = Replace Array Subset(array=w962, new element=w955, index=w952) -> (w969:dbl[])
                                n403 = Replace Array Subset(array=w956, new element=w955, index=w952) -> (w957:dbl[])
                              }
                            }
                          }
                          frame #2 {
                            w983 = 0  # <none>
                            n404 = global write "Global ER2007.vi" "New Setup"(FALSE ("New Setup")) -> ()
                          }
                        }
                      }
                      frame True {
                        # "asserts the TakePt flag"
                        # "Take pt - new volume"
                        n405 = local read "Disp Pv (ml)"() -> (w1004:dbl[])
                        n406 = global read "Global ER2007.vi" "TakePtCell"() -> (w987:i32)
                        n407 = global write "Global ER2007.vi" "TakePt"(FALSE ("New Vol")) -> ()
                        n408 = Unbundle By Name(w996) -> ("Cell Data"=w1016:T6)
                        n409 = Decrement(x=w987) -> (x-1=w986:i32)
                        n410 = Index Array(array=w1016, index=w986) -> (element=w1003:T7)
                        n411 = Unbundle By Name(w1003) -> ("Last Pore Vol"=w991:dbl)
                        n412 = case shown="False" "Defeated" {
                          tunnel: [w1017 w1021] -> w988
                          tunnel: w1004 -> [w1017 w1020]
                          tunnel: w991 -> [_ w1019]
                          tunnel: w986 -> [_ w1018]
                          frame False {
                          }
                          frame True {
                            n413 = Replace Array Subset(array=w1020, new element=w1019, index=w1018) -> (w1021:dbl[])
                          }
                        }
                        n414 = Replace Array Subset(array=w999, new element=TRUE, index=w986) -> (w1000:bool[])
                        n415 = local read "Time"() -> (w1006:timestamp[])
                        n416 = local read "Lapsed Hrs"() -> (w1005:dbl[])
                        n417 = local read "NOP (psig)"() -> (w1008:dbl[])
                        n418 = local read "ER 1-2"() -> (w1014:dbl[])
                        n419 = local read "T-A (°C)"() -> (w1010:dbl[])
                        n420 = local read "T-B (°C)"() -> (w1009:dbl[])
                        n421 = local read "ER 2-3"() -> (w1011:dbl[])
                        n422 = local read "ER 1-3"() -> (w1013:dbl[])
                        n423 = local read "Delta P (psi)"() -> (w989:dbl[])
                        n424 = local read "ER 1-4"() -> (w1012:dbl[])
                        n425 = local read "F 2-3"() -> (w1002:dbl[])
                        n426 = local read "Pc-d(psig)"() -> (w990:dbl[])
                        n427 = local read "Sample ID"() -> (w1015:string[])
                        n428 = local read "Pc (psig)"() -> (w1007:dbl[])
                      }
                    }
                  }
                  frame True {
                    # "New\ndata"
                    n429 = stacked-sequence {
                      seq-local: [w1044 _ _] -> [_ w1053 w1139]
                      seq-local: [w1047 _ _] -> [_ w1067 _]
                      seq-local: [w1046 _ _] -> [_ w1052 w1144]
                      tunnel: w1028 -> [w1049 _ _]
                      tunnel: [_ w1066 _] -> w1043
                      tunnel: [_ w1064 _] -> w1042
                      tunnel: [_ w1063 _] -> w1041
                      tunnel: [_ w1061 _] -> w1040
                      tunnel: [_ w1060 _] -> w1039
                      tunnel: [_ w1058 _] -> w1038
                      tunnel: [_ w1057 _] -> w1037
                      tunnel: [_ w1056 _] -> w1036
                      tunnel: [_ w1055 _] -> w1035
                      tunnel: [_ w1054 _] -> w1034
                      tunnel: [_ w1065 _] -> w1033
                      tunnel: [_ w1062 _] -> w1032
                      tunnel: [_ w1068 _] -> w1031
                      tunnel: [_ w1059 _] -> w1030
                      tunnel: w1029 -> [_ w1068 _]
                      tunnel: [_ _ TRUE] -> w1024
                      tunnel: [_ w1051 _] -> w1023
                      tunnel: [_ w1050 _] -> w1022
                      frame #0 {
                        n430 = global read "Global ER2007.vi" "GCD Err"() -> (w1046:bool)
                        n431 = global read "Global ER2007.vi" "DataCell"() -> (w1045:i32)
                        n432 = Unbundle By Name(w1049) -> ("Cell Data"=w1048:T6)  [unwired: 1 out]
                        n433 = Decrement(x=w1045) -> (x-1=w1044:i32)
                        n434 = Index Array(array=w1048, index=w1044) -> (element=w1047:T7)
                      }
                      frame #1 {
                        n435 = case shown="False" w1052 {
                          tunnel: w1067 -> [w1123 _]
                          tunnel: [w1121 w1138] -> w1066
                          tunnel: [w1075 w1128] -> w1065
                          tunnel: [w1112 w1137] -> w1064
                          tunnel: [w1107 w1136] -> w1063
                          tunnel: [w1104 w1127] -> w1062
                          tunnel: [w1102 w1135] -> w1061
                          tunnel: [w1098 w1134] -> w1060
                          tunnel: [w1096 w1133] -> w1059
                          tunnel: [w1094 w1132] -> w1058
                          tunnel: [w1092 w1131] -> w1057
                          tunnel: [w1086 w1130] -> w1056
                          tunnel: [w1085 w1129] -> w1055
                          tunnel: [w1083 w1126] -> w1054
                          tunnel: w1053 -> [w1074 _]
                          tunnel: [w1077 w1125] -> w1051
                          tunnel: [w1073 w1124] -> w1050
                          frame False {
                            # "No error - update data"
                            n436 = local read "Lapsed Hrs"() -> (w1103:dbl[])
                            n437 = local read "Time"() -> (w1119:timestamp[])
                            n438 = Unbundle By Name(w1123) -> ("Sample #"=w1110:string, "Start Time"=w1079:dbl, "CurData"=w1115:dbl[][])
                            n439 = Get Date/Time In Seconds() -> (seconds since 1Jan1904=w1118:timestamp)
                            n440 = Index Array(array=w1115, index (col)=0 ("disabled index (col)")) -> (element=w1117:dbl[])  [unwired: 1 in]
                            n441 = Array Size(array=w1117) -> (size(s)=w1116:i32)
                            n442 = call "Sample Timer Functions.vi"("Start Time"=w1079) -> ("Elapsed Hours"=w1078:dbl)  [unwired: 5 in, 5 out]
                            n443 = Decrement(x=w1116) -> (x-1=w1109:i32)
                            n444 = Index Array(array=w1115, index (row)=w1109) -> (element=w1114:dbl[])  [unwired: 1 in]
                            n445 = Replace Array Subset(array=w1119, new element=w1118, index=w1074) -> (w1075:timestamp[])
                            n446 = Index Array(array=w1114, index #1=1 ("index")) -> (element #1=w1108:dbl, element #2=w1105:dbl, element #3=w1100:dbl, element #4=w1097:dbl, element #5=w1090:dbl, element #6=w1089:dbl, element #7=w1088:dbl, element #8=w1082:dbl, element #9=w1081:dbl, element #10=w1080:dbl, element #11=w1076:dbl, element #12=w1072:dbl)  [unwired: 11 in]
                            n447 = Replace Array Subset(array=w1103, new element=w1078, index=w1074) -> (w1104:dbl[])
                            n448 = local read "T-A (°C)"() -> (w1093:dbl[])
                            n449 = local read "NOP (psig)"() -> (w1087:dbl[])
                            n450 = local read "Delta P (psi)"() -> (w1071:dbl[])
                            n451 = local read "Disp Pv (ml)"() -> (w1069:dbl[])
                            n452 = local read "ER 1-2"() -> (w1111:dbl[])
                            n453 = local read "T-B (°C)"() -> (w1091:dbl[])
                            n454 = local read "ER 1-4"() -> (w1101:dbl[])
                            n455 = local read "ER 2-3"() -> (w1099:dbl[])
                            n456 = local read "Pc-d(psig)"() -> (w1070:dbl[])
                            n457 = local read "ER 1-3"() -> (w1106:dbl[])
                            n458 = local read "F 2-3"() -> (w1095:dbl[])
                            n459 = local read "Pc (psig)"() -> (w1084:dbl[])
                            n460 = local read "Sample ID"() -> (w1122:string[])
                            n461 = Replace Array Subset(array=w1095, new element=w1090, index=w1074) -> (w1096:dbl[])
                            n462 = Replace Array Subset(array=w1111, new element=w1108, index=w1074) -> (w1112:dbl[])
                            n463 = Replace Array Subset(array=w1091, new element=w1088, index=w1074) -> (w1092:dbl[])
                            n464 = Replace Array Subset(array=w1101, new element=w1100, index=w1074) -> (w1102:dbl[])
                            n465 = Replace Array Subset(array=w1070, new element=w1076, index=w1074) -> (w1077:dbl[])
                            n466 = Replace Array Subset(array=w1084, new element=w1081, index=w1074) -> (w1085:dbl[])
                            n467 = Replace Array Subset(array=w1069, new element=w1072, index=w1074) -> (w1073:dbl[])
                            n468 = Replace Array Subset(array=w1122, new element=w1110, index=w1074) -> (w1121:string[])
                            n469 = Replace Array Subset(array=w1106, new element=w1105, index=w1074) -> (w1107:dbl[])
                            n470 = Replace Array Subset(array=w1099, new element=w1097, index=w1074) -> (w1098:dbl[])
                            n471 = Replace Array Subset(array=w1093, new element=w1089, index=w1074) -> (w1094:dbl[])
                            n472 = Replace Array Subset(array=w1087, new element=w1082, index=w1074) -> (w1086:dbl[])
                            n473 = Replace Array Subset(array=w1071, new element=w1080, index=w1074) -> (w1083:dbl[])
                          }
                          frame True {
                            # "GCD error - don't update"
                            n474 = local read "Lapsed Hrs"() -> (w1127:dbl[])
                            n475 = local read "Delta P (psi)"() -> (w1126:dbl[])
                            n476 = local read "Disp Pv (ml)"() -> (w1124:dbl[])
                            n477 = local read "NOP (psig)"() -> (w1130:dbl[])
                            n478 = local read "Sample ID"() -> (w1138:string[])
                            n479 = local read "Pc-d(psig)"() -> (w1125:dbl[])
                            n480 = local read "Pc (psig)"() -> (w1129:dbl[])
                            n481 = local read "T-A (°C)"() -> (w1132:dbl[])
                            n482 = local read "T-B (°C)"() -> (w1131:dbl[])
                            n483 = local read "ER 1-2"() -> (w1137:dbl[])
                            n484 = local read "ER 2-3"() -> (w1134:dbl[])
                            n485 = local read "ER 1-3"() -> (w1136:dbl[])
                            n486 = local read "ER 1-4"() -> (w1135:dbl[])
                            n487 = local read "F 2-3"() -> (w1133:dbl[])
                            n488 = local read "Time"() -> (w1128:timestamp[])
                          }
                        }
                      }
                      frame #2 {
                        # "Clears flags, updates selected cell status"
                        n489 = case shown="True" w1144 {
                          tunnel: [FALSE ("C1-Status") TRUE ("C1-Status")] -> w1143
                          tunnel: [w1155 w1157] -> w1142
                          frame False {
                            w1155 = cluster{u32, u32}[] [{1985280, 1985280}, {6618880, 6618880}, {1985280, 1985280}, {6618880, 6618880}]  # Busy Colors
                            # "No error"
                          }
                          frame True {
                            w1157 = cluster{u32, u32}[] [{1985280, 1985280}, {15670784, 15670784}, {1985280, 1985280}, {7802624, 7802624}]  # Error Colors
                            # "GCD error"
                          }
                        }
                        n490 = global write "Global ER2007.vi" "New Data"(FALSE ("New Data")) -> ()
                        n491 = case shown="1" w1139 {
                          tunnel: w1143 -> [w1146 w1148 w1150 w1152 w1154]
                          tunnel: w1142 -> [w1145 w1147 w1149 w1151 w1153]
                          frame 0, Default {
                            n492 = property on="C1-Status" class="Bool (strict)"("Value"=w1146, "Colors [4]"=w1145) -> ()  [unwired: 2 in, 2 out]
                          }
                          frame 1 {
                            n493 = property on="C2-Status" class="Bool (strict)"("Value"=w1148, "Colors [4]"=w1147) -> ()  [unwired: 2 in, 2 out]
                          }
                          frame 2 {
                            n494 = property on="C3-Status" class="Bool (strict)"("Value"=w1150, "Colors [4]"=w1149) -> ()  [unwired: 2 in, 2 out]
                          }
                          frame 3 {
                            n495 = property on="C4-Status" class="Bool (strict)"("Value"=w1152, "Colors [4]"=w1151) -> ()  [unwired: 2 in, 2 out]
                          }
                          frame 4 {
                            n496 = property on="C5-Status" class="Bool (strict)"("Value"=w1154, "Colors [4]"=w1153) -> ()  [unwired: 2 in, 2 out]
                          }
                        }
                      }
                    }
                  }
                }
                "Sample ID" <- w823
                "ER 1-2" <- w822
                "ER 1-3" <- w821
                "ER 1-4" <- w820
                "ER 2-3" <- w819
                "T-A (°C)" <- w818
                "T-B (°C)" <- w817
                "NOP (psig)" <- w816
                "Pc (psig)" <- w815
                "Time" <- w814
                "Lapsed Hrs" <- w813
                "Disp Pv (ml)" <- w799
                "F 2-3" <- w812
                "Pc-d(psig)" <- w797
                "Delta P (psi)" <- w798
              }
            }
            "SelCell" <- w492
            "SetupCell" <- w491
          }
          event "Radio Cell Selects": Value Change {
            # "Cell Selects chgd"
            n497 = event-data() -> ("NewVal"=w1167:T2)  [unwired: 1 in]
            n498 = case shown="\"CS 1\", Default" w1167 {
              selector: w1167 -> [_ w1172]
              tunnel: w1164 -> [_ _]
              tunnel: [w1170 w1171] -> w1163
              frame "No Selection" {
                w1170 = 0  # <none>
              }
              frame "CS 1", Default {
                n499 = case shown="\"No Selection\", Default" w1172 {
                  tunnel: [w1173 1 2 3 4 5] -> w1171
                  frame "No Selection", Default {
                    w1173 = 0  # <none>
                  }
                  frame "CS 1" {
                  }
                  frame "CS 2" {
                  }
                  frame "CS 3" {
                  }
                  frame "CS 4" {
                  }
                  frame "CS 5" {
                  }
                }
              }
            }
          }
          event "TakePt": Value Change {
            # "TakePt chgd"
            n500 = event-data() -> ()  [unwired: 1 in, 1 out]
            n501 = stacked-sequence {
              tunnel: w1187 -> [w1190 _]
              frame #0 {
                # "Loads the Cell #"
                n502 = case shown="\"No Selection\", Default" w1190 {
                  tunnel: [0 1 ("Selected Radio Cell") 2 ("Selected Radio Cell") 3 ("Selected Radio Cell") 4 ("Selected Radio Cell") 5 ("Selected Radio Cell")] -> w1189
                  frame "No Selection", Default {
                  }
                  frame "CS 1" {
                  }
                  frame "CS 2" {
                  }
                  frame "CS 3" {
                  }
                  frame "CS 4" {
                  }
                  frame "CS 5" {
                  }
                }
                n503 = global write "Global ER2007.vi" "TakePtCell"(w1189) -> ()
              }
              frame #1 {
                # "Runs the popup panel vi"
                n504 = Open VI Reference(vi path=path "ER2007 Take Data Popup Panel.vi") -> (vi reference=w1204:refnum<vi>, error out=w1203:errorcluster)  [unwired: 5 in]
                n505 = property class="VI"(reference=w1204, error in=w1203, "Front Panel Window:Open"=TRUE) -> (reference out=w1201:refnum<vi>, error out=w1200:errorcluster)
                n506 = invoke class="VI" method="Run VI"(reference=w1201, error in=w1200, "Wait until done"=FALSE, "Auto Dispose Ref"=TRUE) -> (error out=w1197:errorcluster)  [unwired: 1 in, 4 out]
                n507 = call <vilib>:"Simple Error Handler.vi"("error in (no error)"=w1197) -> ()  [unwired: 4 in, 5 out]
              }
            }
          }
          event "Setup": Value Change {
            # "Setup"
            n508 = event-data() -> ()  [unwired: 1 in, 1 out]
            n509 = stacked-sequence {
              tunnel: w1214 -> [w1217 _]
              tunnel: [w1216 _] -> w1210
              frame #0 {
                n510 = case shown="\"No Selection\", Default" w1217 {
                  tunnel: [0 1 ("Selected Radio Cell") 2 ("Selected Radio Cell") 3 ("Selected Radio Cell") 4 ("Selected Radio Cell") 5 ("Selected Radio Cell")] -> w1216
                  frame "No Selection", Default {
                  }
                  frame "CS 1" {
                  }
                  frame "CS 2" {
                  }
                  frame "CS 3" {
                  }
                  frame "CS 4" {
                  }
                  frame "CS 5" {
                  }
                }
                n511 = global write "Global ER2007.vi" "New Setup"(FALSE ("New Setup")) -> ()
                n512 = global write "Global ER2007.vi" "SetupCell"(w1216) -> ()
              }
              frame #1 {
                # "Launches Test Def Panel (Setup)"
                n513 = Open VI Reference(vi path=path "ER2007 Test Definition Panel.vi") -> (vi reference=w1232:refnum<vi>, error out=w1231:errorcluster)  [unwired: 5 in]
                n514 = property class="VI"(reference=w1232, error in=w1231, "Front Panel Window:Open"=TRUE) -> (reference out=w1229:refnum<vi>, error out=w1228:errorcluster)
                n515 = invoke class="VI" method="Run VI"(reference=w1229, error in=w1228, "Wait until done"=FALSE, "Auto Dispose Ref"=TRUE) -> (error out=w1225:errorcluster)  [unwired: 1 in, 4 out]
                n516 = call <vilib>:"Simple Error Handler.vi"("error in (no error)"=w1225) -> ()  [unwired: 4 in, 5 out]
              }
            }
          }
          event "History": Value Change {
            # "History"
            n517 = event-data() -> ()  [unwired: 1 in, 1 out]
            n518 = stacked-sequence {
              tunnel: w1242 -> [w1245 _]
              frame #0 {
                n519 = case shown="\"No Selection\", Default" w1245 {
                  tunnel: [0 1 ("Selected Radio Cell") 2 ("Selected Radio Cell") 3 ("Selected Radio Cell") 4 ("Selected Radio Cell") 5 ("Selected Radio Cell")] -> w1244
                  frame "No Selection", Default {
                  }
                  frame "CS 1" {
                  }
                  frame "CS 2" {
                  }
                  frame "CS 3" {
                  }
                  frame "CS 4" {
                  }
                  frame "CS 5" {
                  }
                }
                n520 = global write "Global ER2007.vi" "SetupCell"(w1244) -> ()
              }
              frame #1 {
                n521 = Open VI Reference(vi path=path "ER2007 Data History Panel.vi") -> (vi reference=w1259:refnum<vi>, error out=w1258:errorcluster)  [unwired: 5 in]
                n522 = property class="VI"(reference=w1259, error in=w1258, "Front Panel Window:Open"=TRUE) -> (reference out=w1256:refnum<vi>, error out=w1255:errorcluster)
                n523 = invoke class="VI" method="Run VI"(reference=w1256, error in=w1255, "Wait until done"=FALSE, "Auto Dispose Ref"=TRUE) -> (error out=w1252:errorcluster)  [unwired: 1 in, 4 out]
                n524 = call <vilib>:"Simple Error Handler.vi"("error in (no error)"=w1252) -> ()  [unwired: 4 in, 5 out]
              }
            }
          }
          event "CurVals": Value Change {
            # "Current values"
            n525 = event-data() -> ()  [unwired: 1 in, 1 out]
            n526 = Open VI Reference(vi path=path "ER2007 Current Values Panel.vi") -> (vi reference=w1276:refnum<vi>, error out=w1275:errorcluster)  [unwired: 5 in]
            n527 = property class="VI"(reference=w1276, error in=w1275, "Front Panel Window:Open"=TRUE) -> (reference out=w1273:refnum<vi>, error out=w1272:errorcluster)
            n528 = invoke class="VI" method="Run VI"(reference=w1273, error in=w1272, "Wait until done"=FALSE, "Auto Dispose Ref"=TRUE) -> (error out=w1269:errorcluster)  [unwired: 1 in, 4 out]
            n529 = call <vilib>:"Simple Error Handler.vi"("error in (no error)"=w1269) -> ()  [unwired: 4 in, 5 out]
          }
          event "Utilities": Value Change {
            # "Utilities"
            n530 = event-data() -> ()  [unwired: 1 in, 1 out]
            n531 = Open VI Reference(vi path=path "ER2007 Password Popup Panel.vi") -> (vi reference=w1297:refnum<vi>, error out=w1296:errorcluster)  [unwired: 5 in]
            n532 = property class="VI"(reference=w1297, error in=w1296, "Front Panel Window:Open"=TRUE) -> (reference out=w1294:refnum<vi>, error out=w1293:errorcluster)
            n533 = invoke class="VI" method="Run VI"(reference=w1294, error in=w1293, "Wait until done"=FALSE, "Auto Dispose Ref"=TRUE) -> (error out=w1290:errorcluster)  [unwired: 1 in, 4 out]
            n534 = call <vilib>:"Simple Error Handler.vi"("error in (no error)"=w1290) -> ()  [unwired: 4 in, 5 out]
          }
          event "Reset DAQ": Value Change {
            # "Reset DAQ"
            n535 = event-data() -> ("NewVal"=w1301:bool)  [unwired: 1 in]
            n536 = case shown="True" w1301 {
              frame False {
              }
              frame True {
                n537 = global write "Global ER2007.vi" "DAQ Init"(TRUE) -> ()
              }
            }
          }
          event "Stop": Value Change {
            # "Stop"
            n538 = event-data() -> ()  [unwired: 1 in, 1 out]
            n539 = stacked-sequence {
              frame #0 {
                n540 = global write "Global ER2007.vi" "STOP Done"(FALSE ("STOP Done")) -> ()
              }
              frame #1 {
                n541 = Open VI Reference(vi path=path "ER2007 Are You Sure Popup Panel.vi") -> (vi reference=w1329:refnum<vi>, error out=w1328:errorcluster)  [unwired: 5 in]
                n542 = property class="VI"(reference=w1329, error in=w1328, "Front Panel Window:Open"=TRUE) -> (reference out=w1326:refnum<vi>, error out=w1325:errorcluster)
                n543 = invoke class="VI" method="Run VI"(reference=w1326, error in=w1325, "Wait until done"=FALSE, "Auto Dispose Ref"=TRUE) -> (error out=w1322:errorcluster)  [unwired: 1 in, 4 out]
                n544 = call <vilib>:"Simple Error Handler.vi"("error in (no error)"=w1322) -> ()  [unwired: 4 in, 5 out]
              }
            }
          }
        }
        "Status" <- w472
        "Refresh" <- w460
        "Schd Times" <- w468
        "GCDCell" <- w464
      }
    }
    frame #2 {
      # "Cleanup and shutdown"
      n545 = stacked-sequence {
        tunnel: w1331 -> [w1335 _ _]
        frame #0 {
          w1332 = FALSE ("Visible")
          w1334 = TRUE  # Stop
          w1337 = FALSE ("C1-Status")
          w1333 = FALSE ("A/D Run")
          w1338 = u8 0 ("Disabled")
          # "Clears variables and properties"
          n546 = global write "Global ER2007.vi" "SysRun"(FALSE ("SysRun")) -> ()
          n547 = local write "Status"(bool[] [FALSE, FALSE, FALSE, FALSE, FALSE] ("Status")) -> ()
          n548 = property on="TakePt" class="Bool"("Disabled"=w1338) -> ()  [unwired: 2 in, 2 out]
          n549 = property on="System Error" class="Bool (strict)"("Visible"=w1332) -> ()  [unwired: 2 in, 2 out]
          n550 = local write "DAQ Run"(w1333) -> ()
          n551 = local write "Radio Cell Selects"(T1."No Selection" ("Radio Cell Selects")) -> ()
          n552 = call "Sample Request Control.vi"("SimOn"=w1335, "Stop"=w1334) -> ()  [unwired: 12 in, 6 out]
          n553 = property on="Setup" class="Bool"("Disabled"=w1338) -> ()  [unwired: 2 in, 2 out]
          n554 = property on="Reset DAQ" class="Bool"("Visible"=w1332) -> ()  [unwired: 2 in, 2 out]
          n555 = local write "A/D Err"(w1333) -> ()
          n556 = property on="History" class="Bool"("Disabled"=w1338) -> ()  [unwired: 2 in, 2 out]
          n557 = local write "GCD Busy"(w1333) -> ()
          n558 = property on="CurVals" class="Bool"("Disabled"=w1338) -> ()  [unwired: 2 in, 2 out]
          n559 = local write "GCD Err"(w1333) -> ()
          n560 = local write "VPA Err"(w1333) -> ()
          "C1-Status" <- w1337
          "C2-Status" <- w1337
          "C3-Status" <- w1337
          "C4-Status" <- w1337
          "C5-Status" <- w1337
        }
        frame #1 {
          # "Waits for Get Cell Data to Stop"
          n561 = Get Date/Time In Seconds() -> (seconds since 1Jan1904=w1342:timestamp)
          n562 = To Double Precision Float(number=w1342) -> (double precision float=w1341:dbl)
          n563 = while {
            tunnel: w1341 -> [w1348]
            stop <- w1346 continue-if-true
            w1347 = 8.0  # T/O = 8 sec
            n564 = Get Date/Time In Seconds() -> (seconds since 1Jan1904=w1350:timestamp)
            n565 = To Double Precision Float(number=w1350) -> (double precision float=w1349:dbl)
            n566 = Subtract(x=w1349, y=w1348) -> (x-y=w1344:dbl)
            n567 = Wait Until Next ms Multiple(millisecond multiple=u32 300) -> ()  [unwired: 1 out]
            n568 = global read "Global ER2007.vi" "GCD Stop"() -> (w1343:bool)
            n569 = Less?(x=w1344, y=w1347) -> (x < y?=w1345:bool)
            n570 = And(x=w1345, y=w1343) -> (x .and. y?=w1346:bool)
          }
        }
        frame #2 {
          # "Exits to LabVIEW or Windows"
          n571 = global read "Global ER2007.vi" "Quit2LV"() -> (w1352:bool)
          n572 = Not(x=w1352) -> (.not. x?=w1353:bool)
          n573 = Quit LabVIEW(quit? (T)=w1353) -> ()
        }
      }
    }
  }
